vi "Panorama Generation- cameras.vi"() -> ()   [LabVIEW 2023]
uses:
  <vilib>/vision/Image Controls.llb/IMAQ Image.ctl
  <vilib>/userDefined/High Color/IMAQdx.ctl
  <vilib>/vision/driver/IMAQdx.llb/IMAQdx Acquisition Mode.ctl
  <vilib>/vision/Calibration.llb/Distortion Model.ctl
  <vilib>/vision/Calibration.llb/Distortion Model Types.ctl
  <vilib>/vision/driver/IMAQdx.llb/IMAQdx Buffer Number Mode.ctl
  <vilib>/vision/EDVR.llb/IMAQ ImageToEDVR 2D SGL.vi
  <vilib>/vision/EDVR.llb/IMAQ ImageToEDVR 2D U8.vi
  <vilib>/vision/NI_Vision_Development_Module.lvlib
  <vilib>/vision/driver/NI_Vision_Acquisition_Software.lvlib
panel:
  in  "?":T1(tab)
  in  "?":enum32{"Processing Time  Display Tab"}(tab)
  out "SSIM Flat":dbl
  out "SSIM Original":dbl
  out "Correction":dbl
  out "Flat Fielding":dbl
  out "ROI Blending":dbl
  out "Processed FPS":dbl
  in  "Stop":bool
  out "Original Luma?":bool
  out "Left corrected, adjusted, and wrapped image":T2(plugin-control) caption="Thresholded Grid"
  out "Right corrected, adjusted, and wrapped image":T2(plugin-control) caption="Thresholded Grid"
  out "Right Sample":T2(plugin-control) caption="Thresholded Grid"
  out "Left Sample":T2(plugin-control) caption="Thresholded Grid"
  out "Panorama Image":T2(plugin-control)
  in  "?":enum32{"Tunning Control Tab"}(tab)
  in  "Wrapping Factor":i32=5
  in  "Correction Interpolation":u32(ring) items=["Zero Order", "Bi-Linear", "Quadratic", "Cubic Spline"]
  in  "Grid Path":path
  in  "Blending Method":enum16{"WA", "MBB", "WE"}(ring)
  in  "Grid Name":string="grid.png"
  in  "ROI_X":i32=10
  in  "Camera 1":T3
  in  "Camera 2":T3
  out "Right corrected, adjusted, and wrapped grid":T2(plugin-control) caption="Right  corrected wrapped grid"
  out "Left corrected, adjusted, and wrapped grid":T2(plugin-control) caption="Left corrected  and wrapped grid"
  out "Thresholded and filtered grid":T2(plugin-control) caption="Thresholded Grid"
  out "Grid Image":T2(plugin-control) caption="Circular Dotted Grid"
  out "ROI_L":T2(plugin-control)
  out "ROI_R":T2(plugin-control)
  out "Blended ROI":T2(plugin-control)
  out "Wrapped Y":i32
  out "Grid X":i32
  out "Grid Y":i32
  out "corrected":T2[](array[typedef])
  out "Adjusted":T2[](array[typedef])
  out "RGB Left":T2[](array[typedef])
  out "RGB Right":T2[](array[typedef])
  out "Y0":dbl
  out "X0":dbl
  out "Y1":dbl
  out "X1":dbl
  out "Y2":dbl
  out "X2":dbl
  out "Wrapped X":i32
  out "GP":T2[][](array[typedef])
  out "LP":T2[][](array[typedef])
  out "Masked RGB Right MBB":T2[](array[typedef])
  out "Masked RGB Left MBB":T2[](array[typedef])
  out "Combined Laplace":T2[][](array[typedef])
  out "Start Time":dbl
  out "Correction End Time":dbl
  out "Flat Fielding End Time":dbl
  out "Blending End Time":dbl
  out "Wrapped":T2[](array[typedef])
  out "error out":errorcluster
  out "corrected size":cluster{"X Resolution":i32, "Y Resolution":i32}
  # "This VI meticulously generates panoramic images through a carefully structured process:\n\nLens Distortion Correction: Specifically addressing Barrel Distortion to ensure precise visual accuracy.\nBrightness Variation Compensation: Achieving a seamless transition by compensating variations in brightness.\nROI Blending: Merging carefully determined Regions of Interest (ROIs) using a selected method (Weighted Average - Default, Multi-Band Blending, Wavelet Extraction).\nFinal Panorama Output: Projecting the corrected and blended elements to produce the ultimate panorama.\n\nUser Steps: Navigate to the \"Tuning Control Tab\" and follow these steps:\n\nSelect Grid Image Path: Specify the path for the grid image.\nInput Grid Image Name: Enter the grid image name as saved in the device, including its extension.\nChoose Left and Right Cameras: Indicate the cameras for the left and right images.\nCorrection Interpolation Type: Determine the interpolation type for the correction process (Zero-Order, or Bilinear).\nSet Wrapping Factor: Define the wrapping factor based on the angle between the cameras.\nROI Resolution: Specify the resolution for the Regions of Interest (ROIs).\nBlending Method: Select the preferred blending method (Weighted Average - Default, Multi-Band Blending, Wavelet Extraction).\nRun the VI."
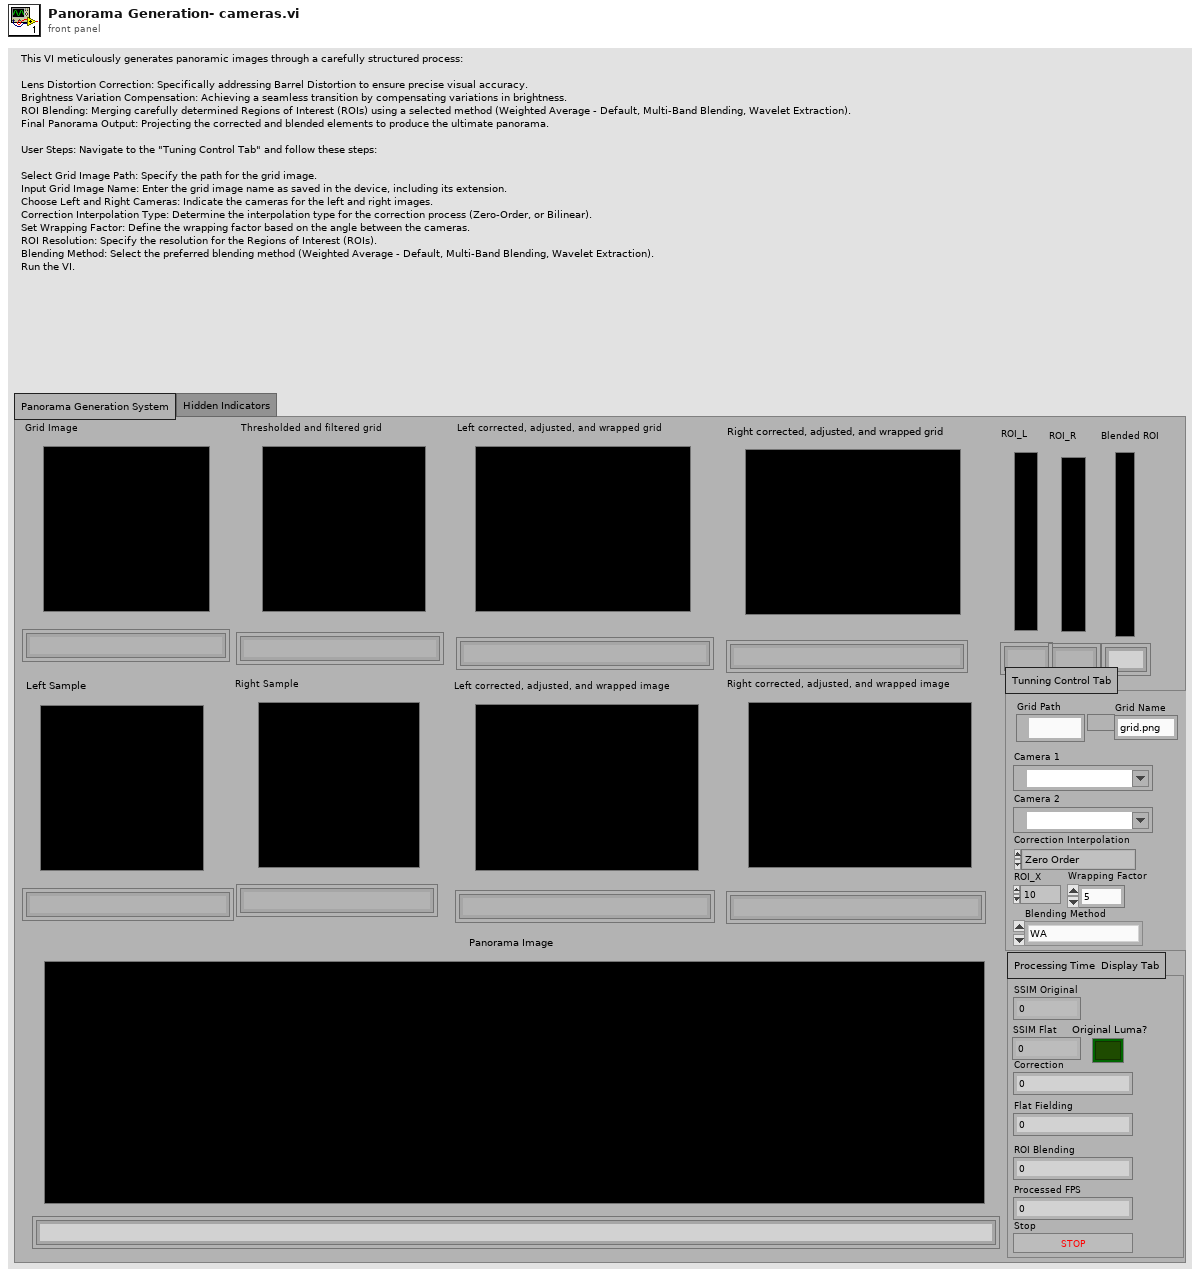
[diagram p1: front panel]
types:
  T1 = enum32{"Panorama Generation System", "Hidden Indicators"}
  T2 = typedef "IMAQ Image.ctl" = refnum<image>
  T3 = typedef "IMAQdx.ctl" = refnum<k21>
  T4 = typedef "NI_Vision_Acquisition_Software.lvlib/IMAQdx Acquisition Mode.ctl" = enum32{"One Shot", "Continuous"}
  T5 = typedef "Image Unit" = enum32{"Undefined", "Angström", "Micrometer", "Millimeter", "Centimeter", "Meter", "Kilometer", "Microinch", "Inch", "Feet", "Nautical miles", "Standard miles", "Steps"}
  T6 = typedef "Particle Parameters" = i32
  T7 = cluster{"Measurement Parameter":T6, "Range Lower Value":dbl, "Range Upper Value":dbl, "Range":bool, "Measurement Type":bool}[]
  T8 = cluster{"Corrected Image Scaling":u32, "Corrected Image Learn ROI":u32, "Learn Correction Table?":bool}
  T9 = typedef "Distortion Model.ctl" = cluster{"Distortion Model":T10, "Polynomial Model Setup":cluster{"Radial Coefficient":u32, "Tangential Coefficients ":bool}}
  T10 = typedef "Distortion Model Types.ctl" = i32
  T11 = typedef "Image Type" = u32
  T12 = typedef "Calibration Reference Points.ctl" = cluster{"Pixel Coordinates":cluster{"X":dbl, "Y":dbl}[], "Real World Coordinates":cluster{"X":dbl, "Y":dbl}[], "Unit":T5, "Image Size":cluster{"X":u32, "Y":u32}}
  T13 = cluster{cluster{"element":dbl, "element":dbl}[], cluster{"element":dbl, "element":dbl}[], "Unit":T5, cluster{"X Resolution":i32, "Y Resolution":i32}}
  T14 = typedef "NI_Vision_Acquisition_Software.lvlib/IMAQdx Buffer Number Mode.ctl" = enum32{"Next", "Last", "Buffer Number", "Every", "Last New"}
  T15 = cluster{"Model":i32, "corrected size":cluster{"X Resolution":i32, "Y Resolution":i32}, "Polynomial Degree":i32}
  T16 = cluster{"Estimate Background?":bool, "Method":i32, "Polynomial Degree":i32, "corrected size":cluster{"X Resolution":i32, "Y Resolution":i32}, "Niblack Deviation Factor (0.2)":dbl}
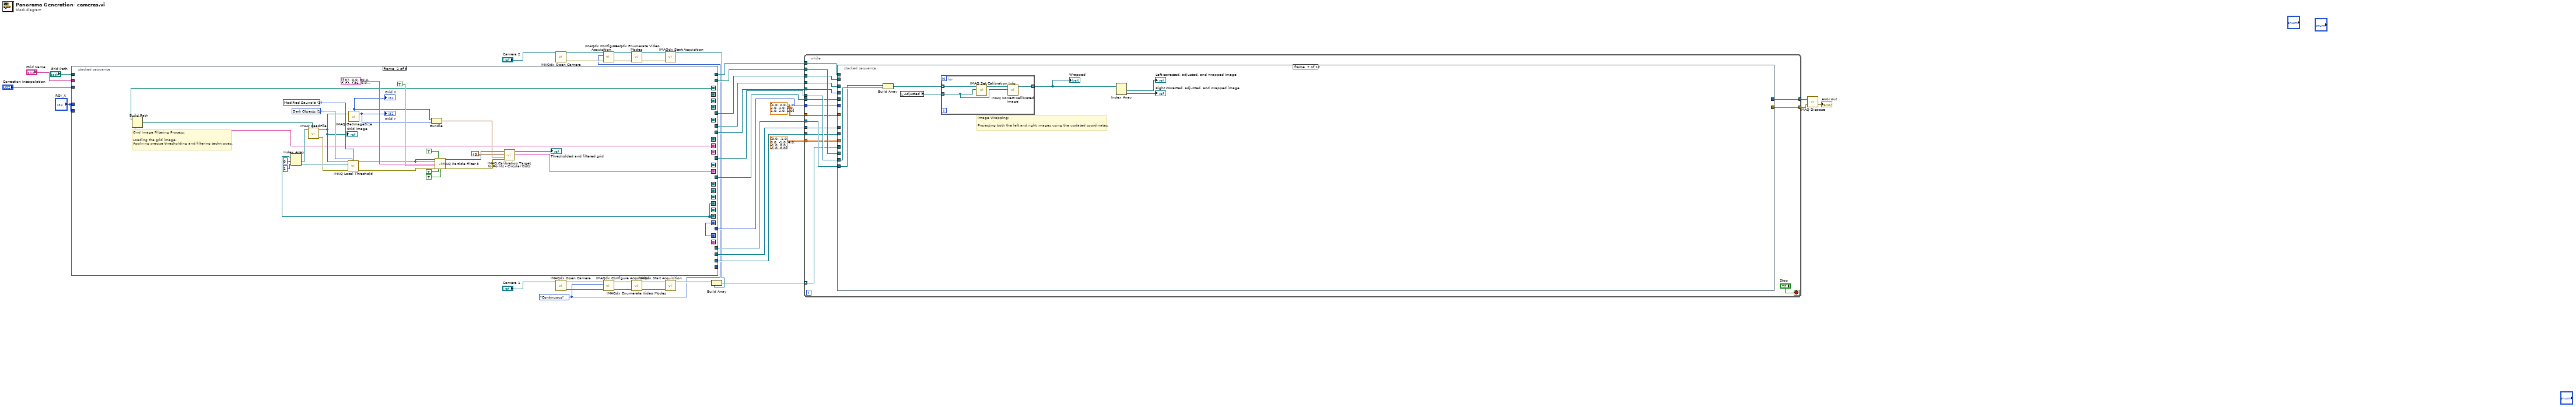
[diagram p0: block diagram]
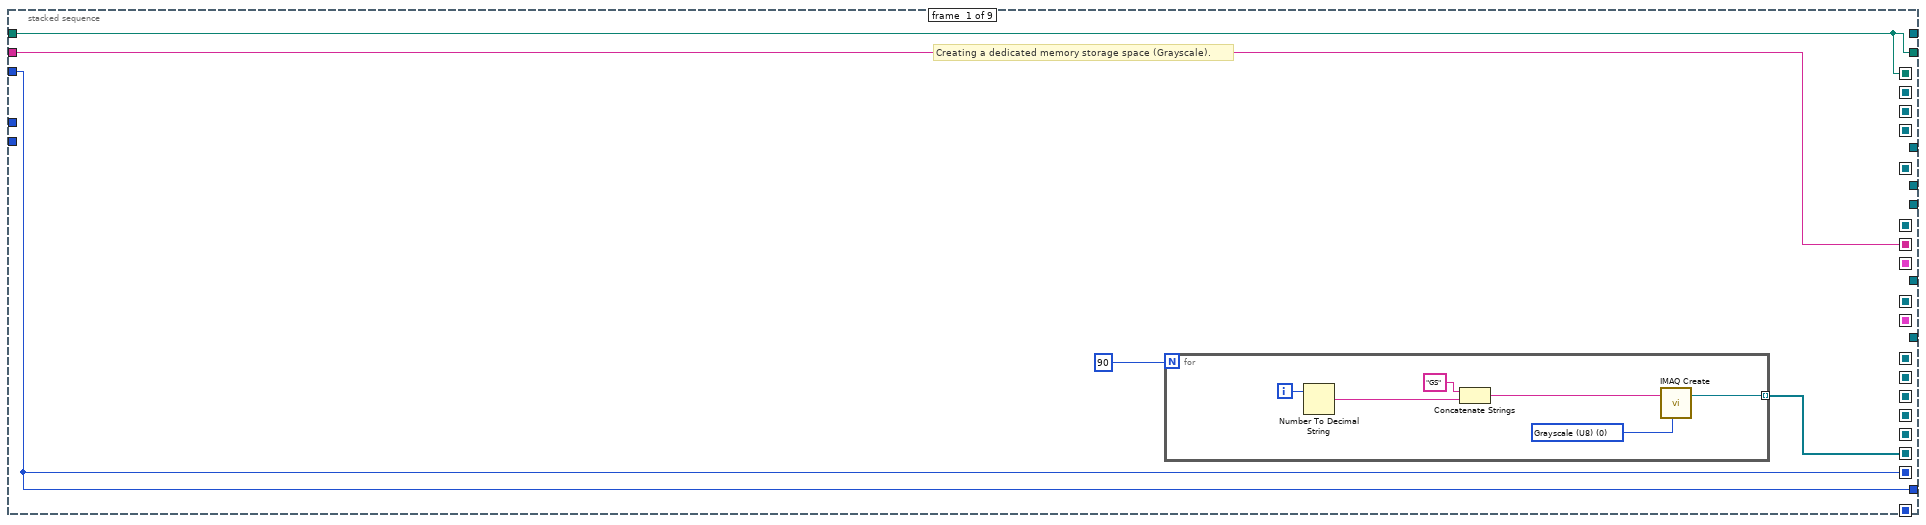
[diagram p2: hidden frame]
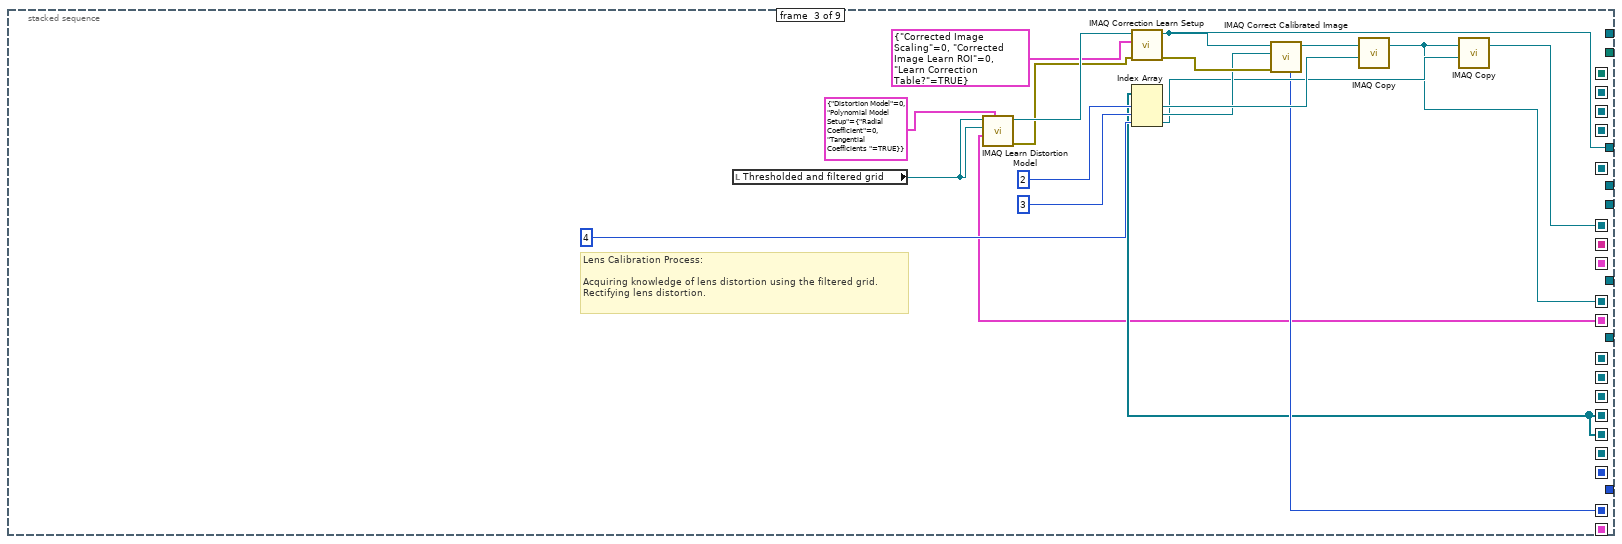
[diagram p3: hidden frame]
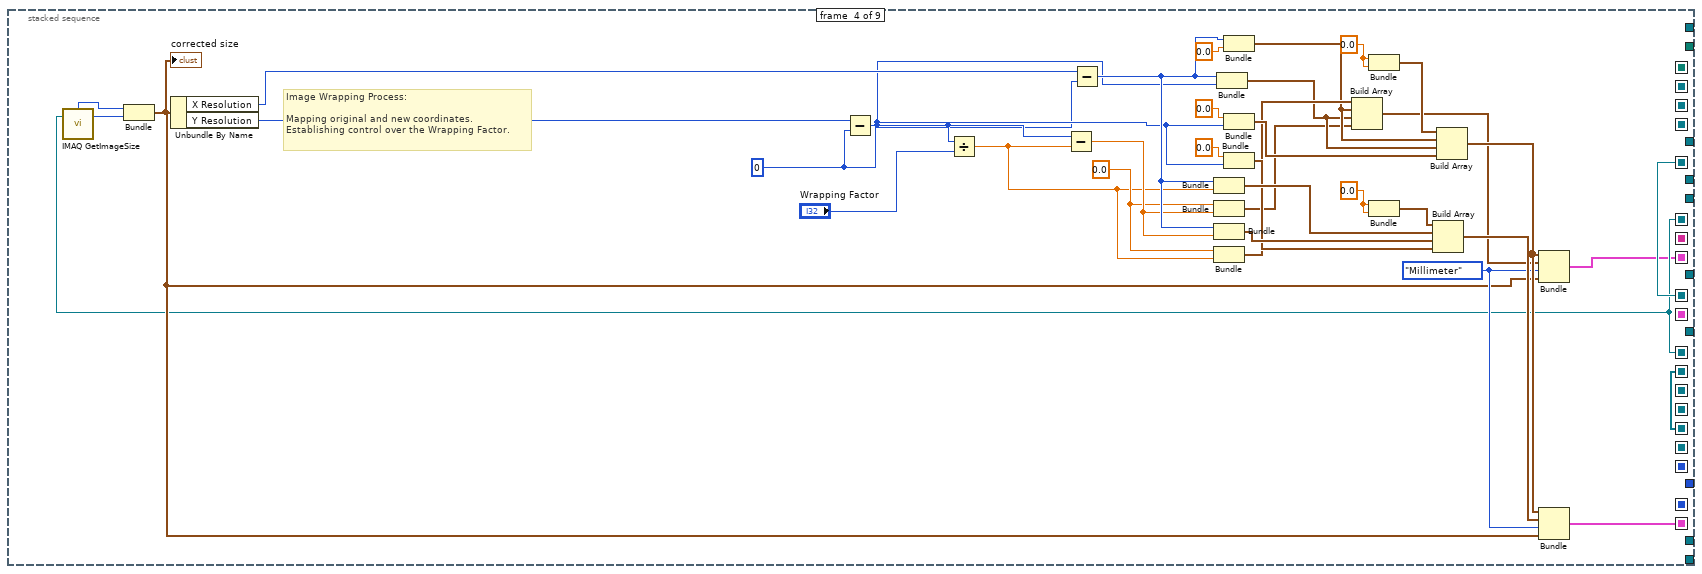
[diagram p4: hidden frame]
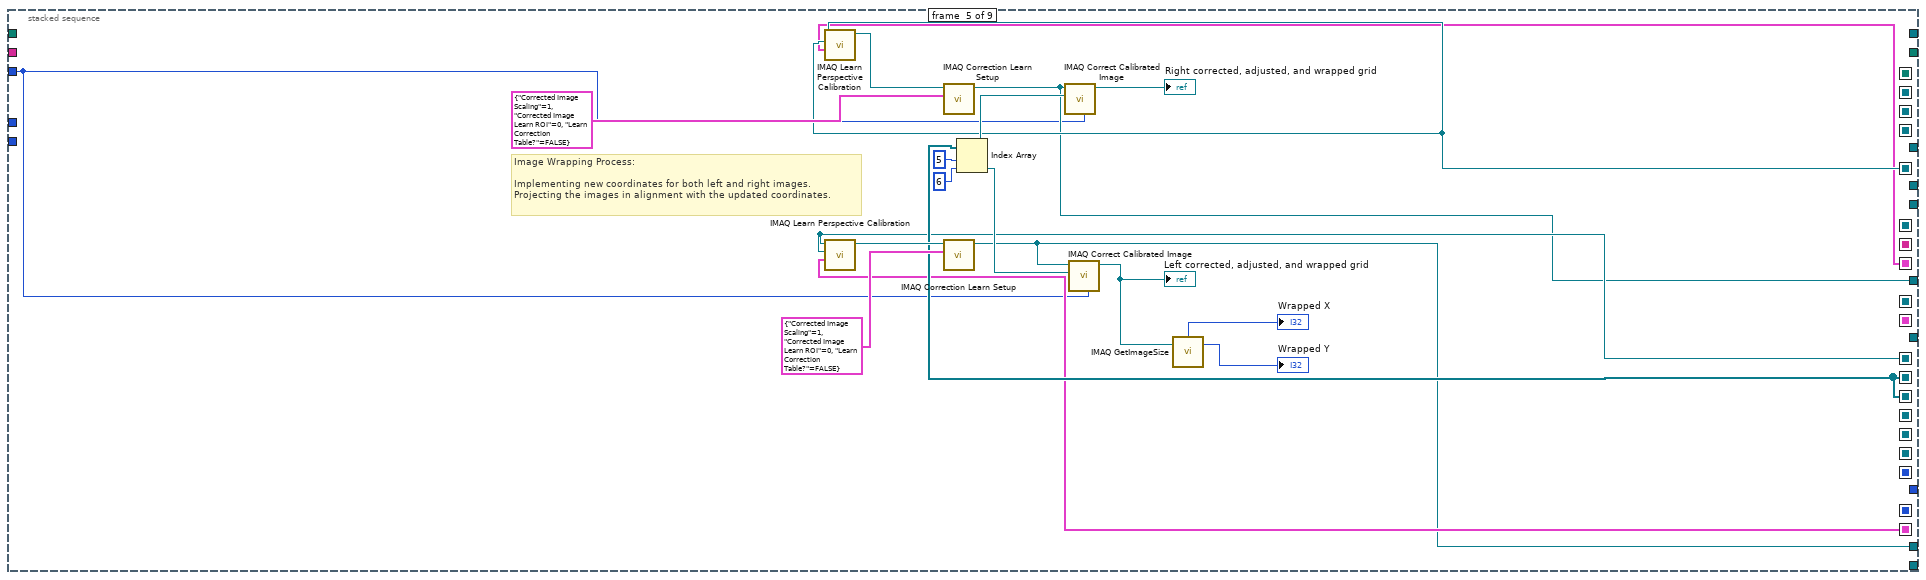
[diagram p5: hidden frame]
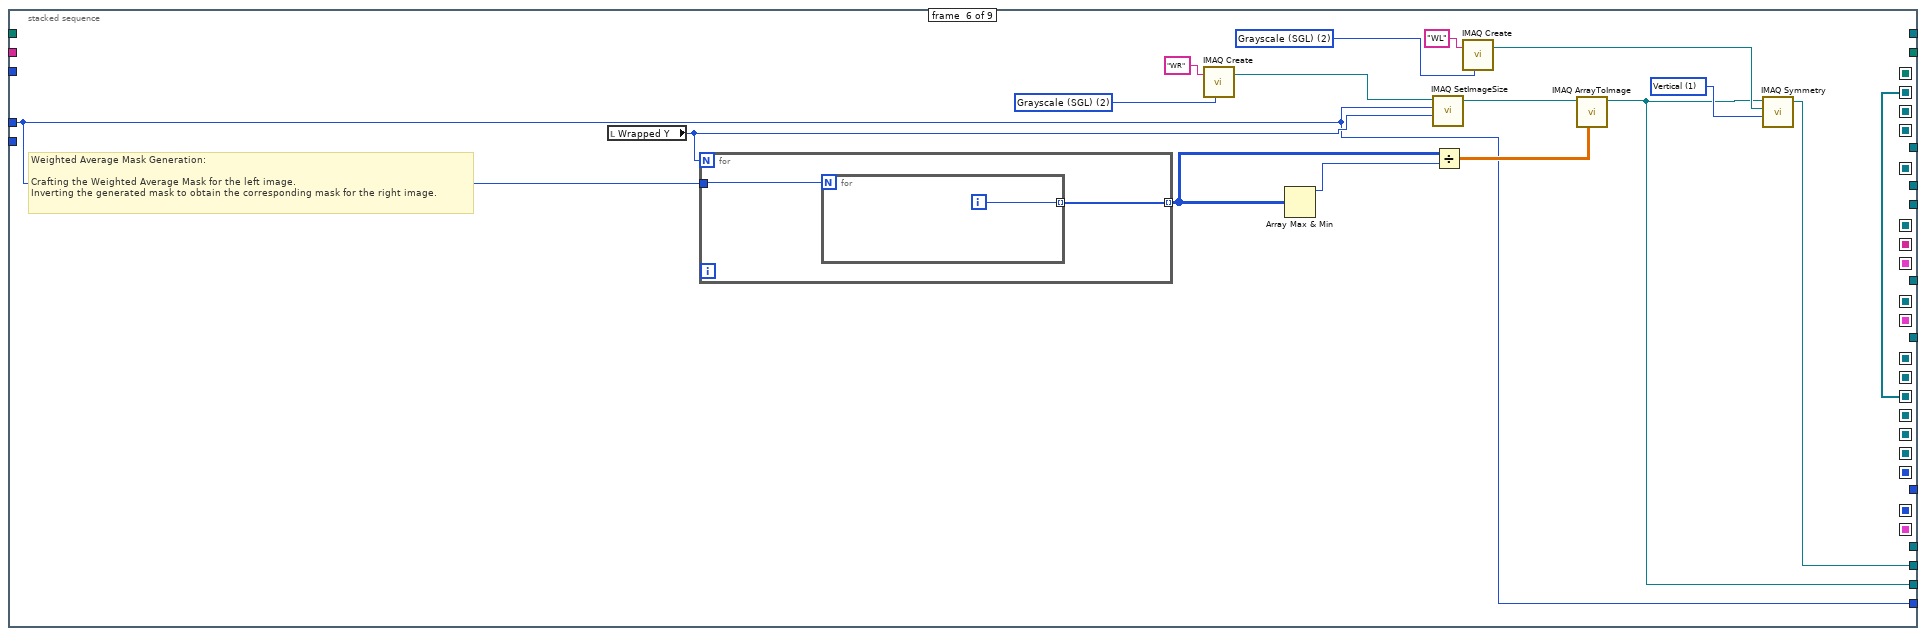
[diagram p6: hidden frame]
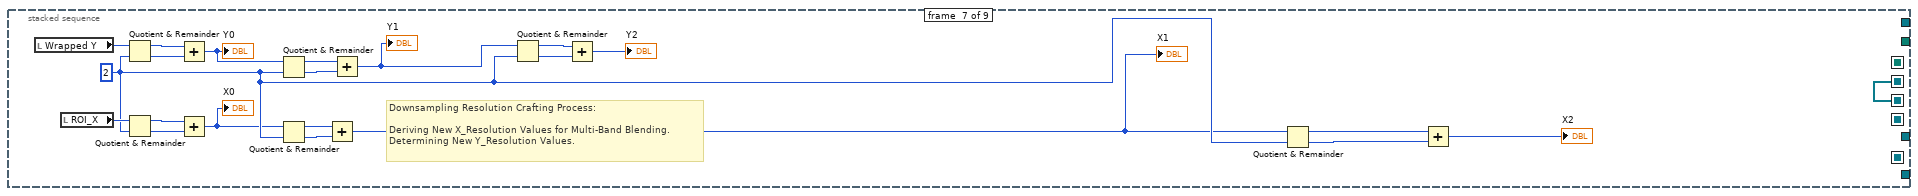
[diagram p7: hidden frame]
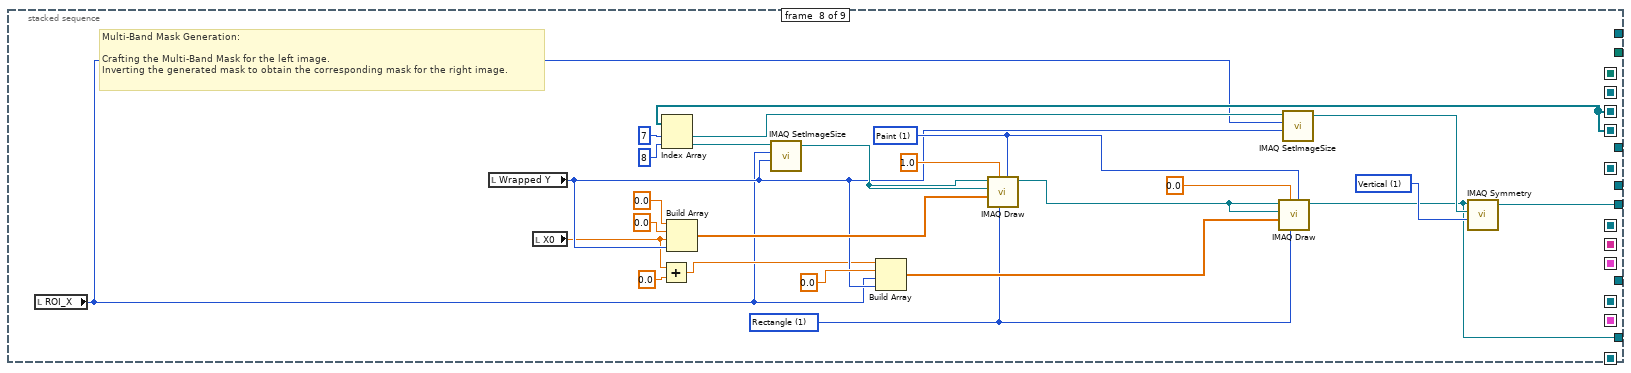
[diagram p8: hidden frame]
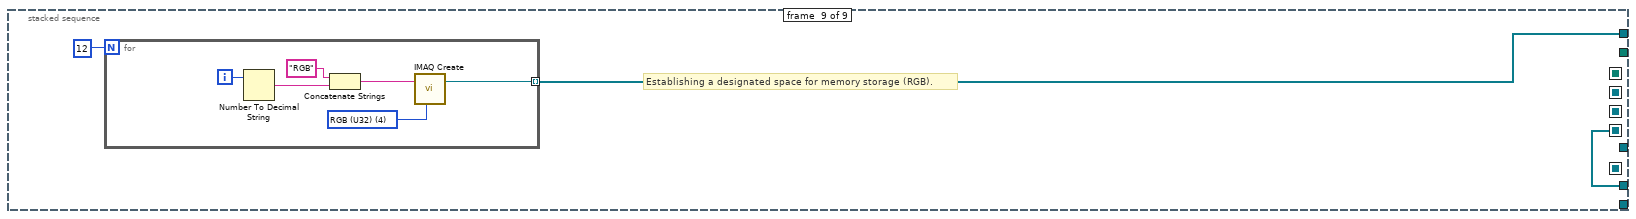
[diagram p9: hidden frame]
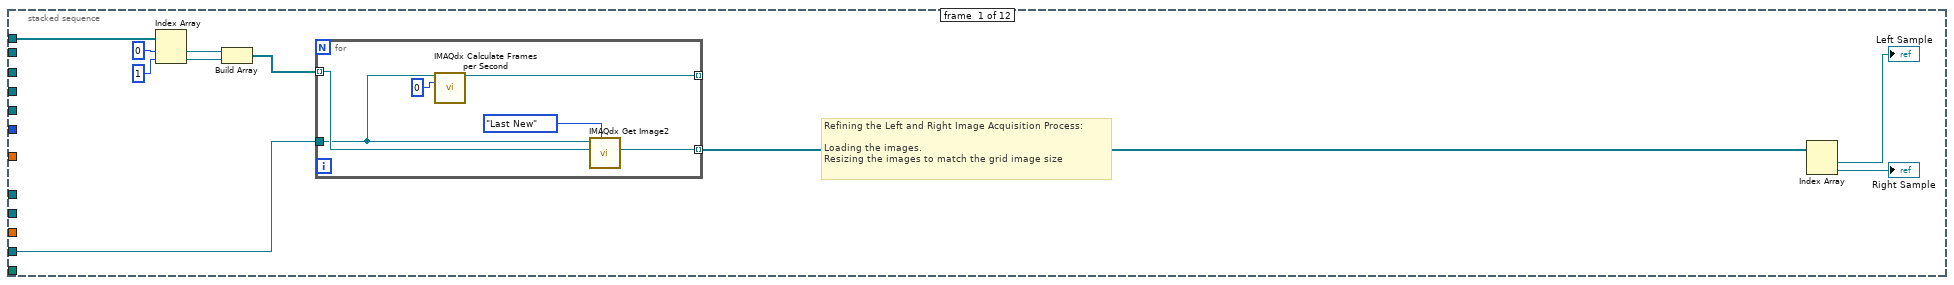
[diagram p10: hidden frame]
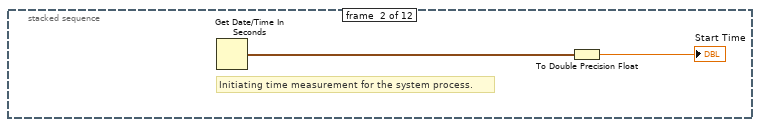
[diagram p11: hidden frame]
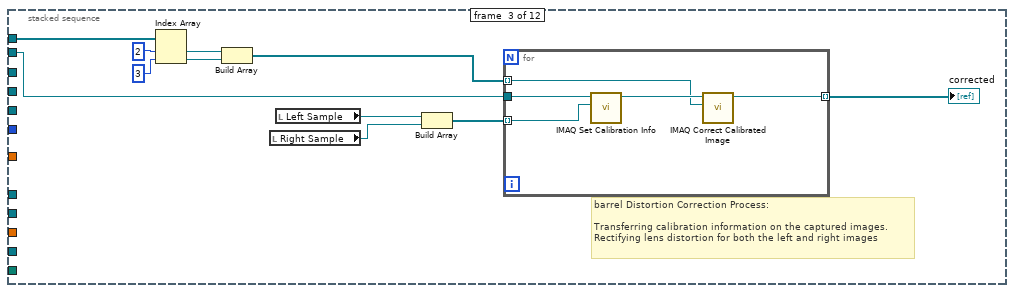
[diagram p12: hidden frame]
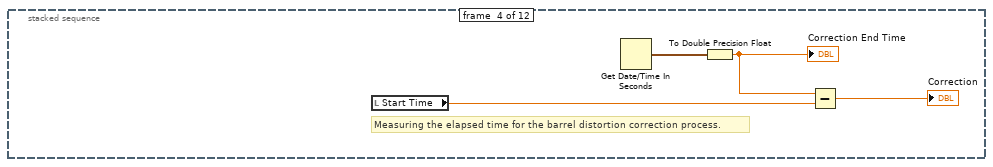
[diagram p13: hidden frame]
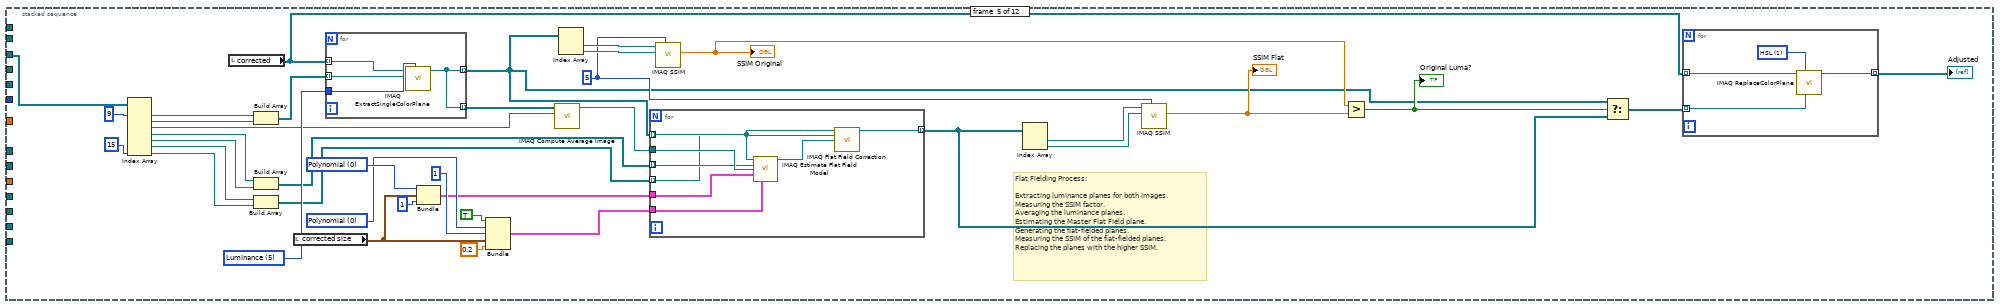
[diagram p14: hidden frame]
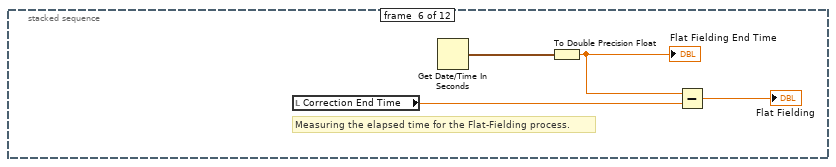
[diagram p15: hidden frame]
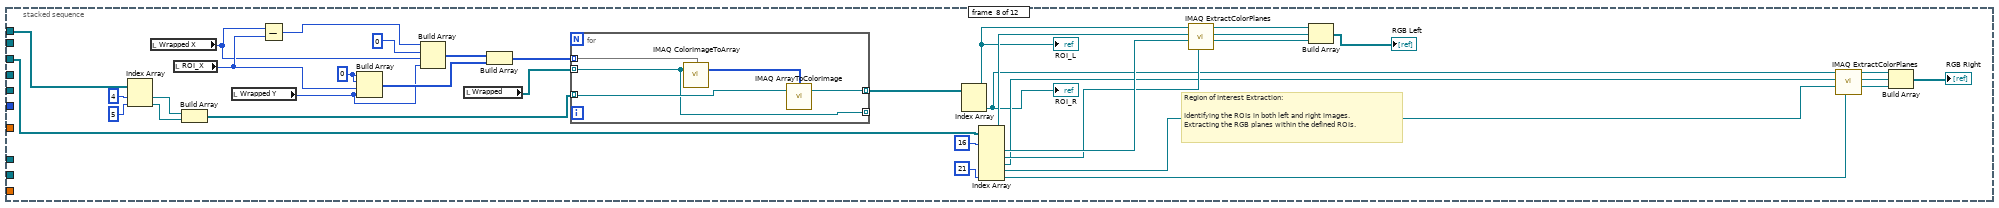
[diagram p16: hidden frame]
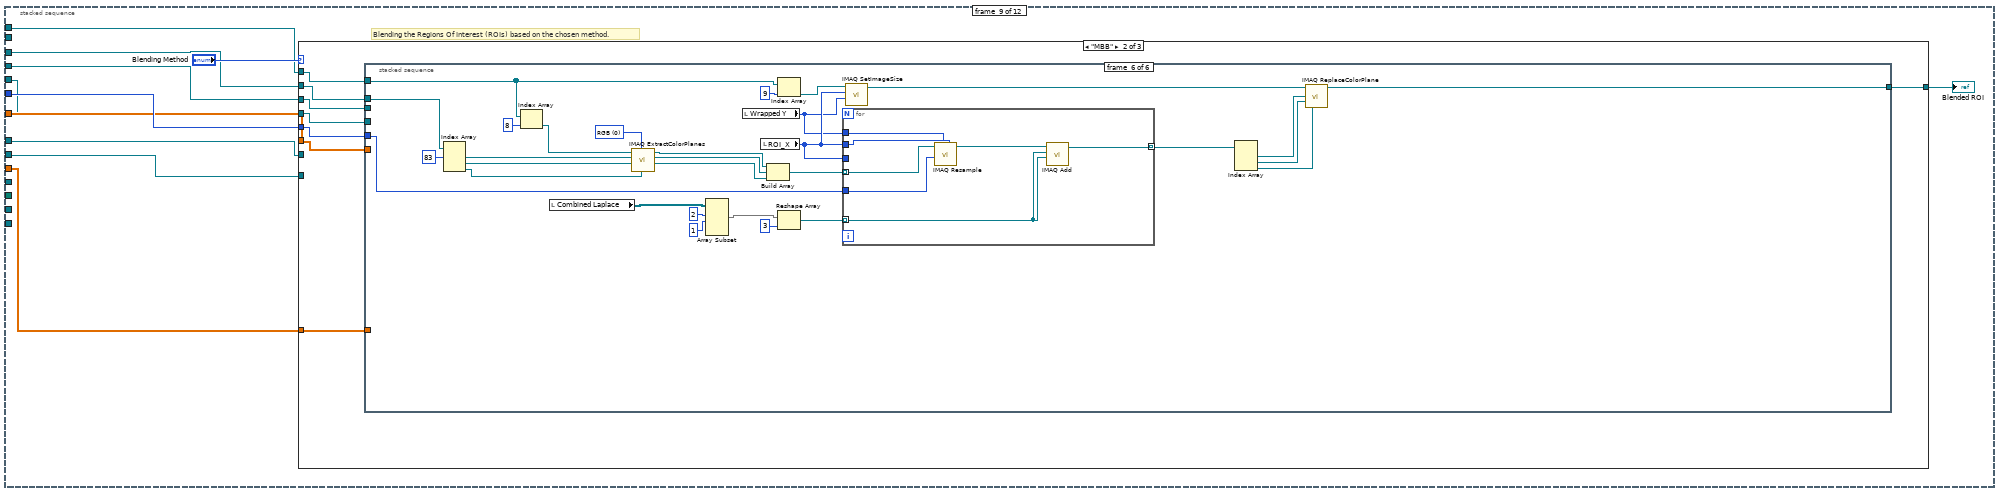
[diagram p17: hidden frame]
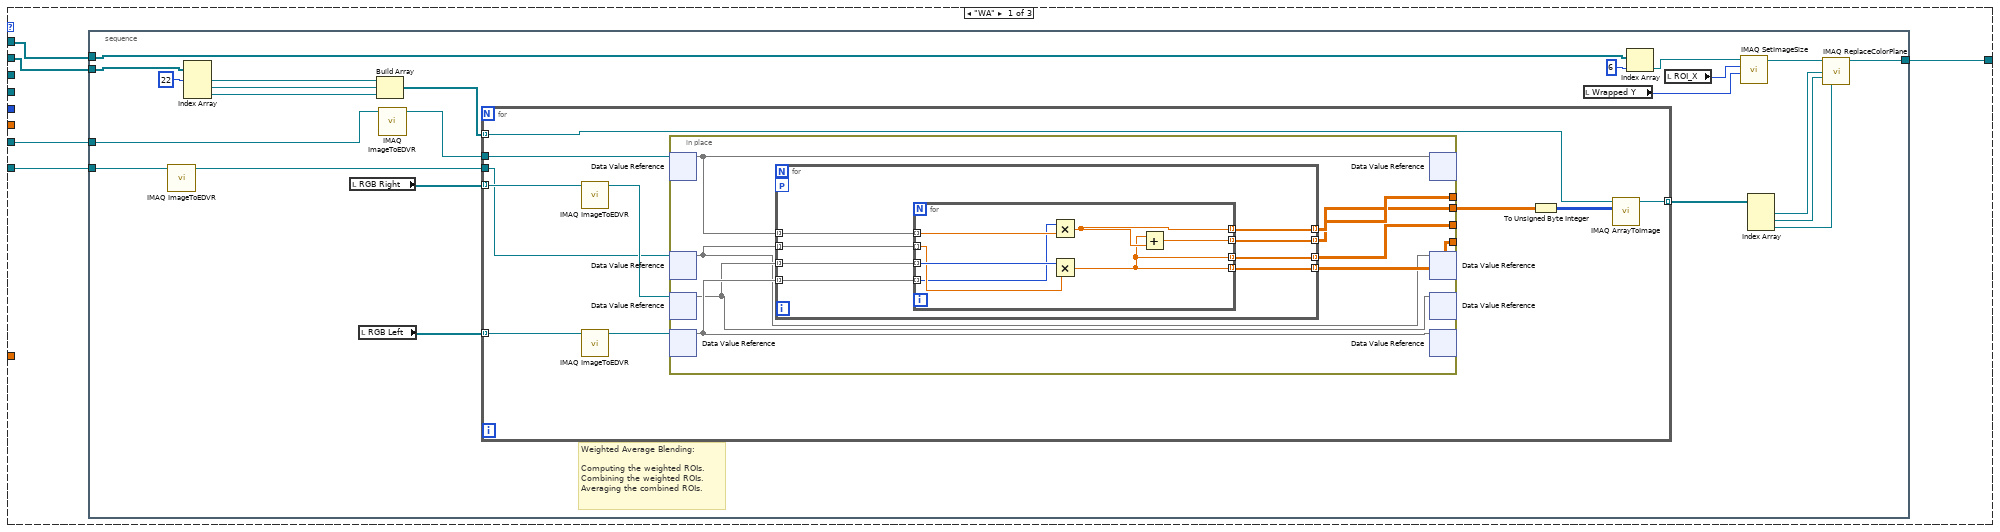
[diagram p18: hidden frame]
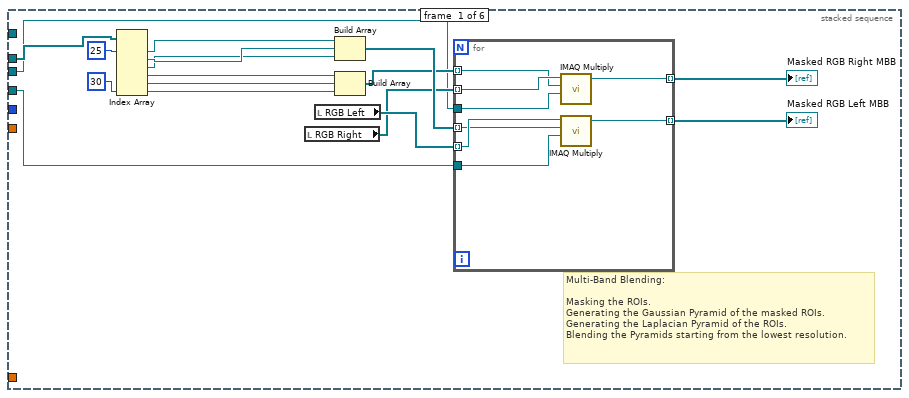
[diagram p19: hidden frame]
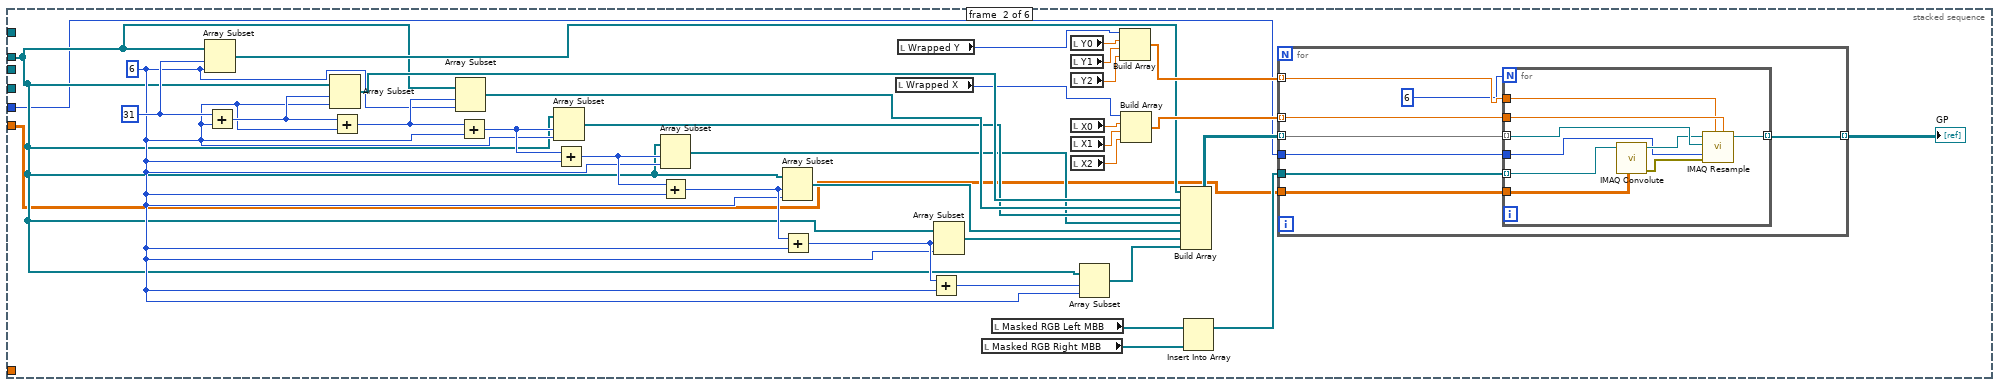
[diagram p20: hidden frame]
diagram:
  w2 = IMAQdx_Acquisition_Mode."Continuous" ("Continuous?")
  n1 = stacked-sequence {
    seq-local: [w40 _ _ _ _ _ _ _ _] -> [_ w56 _ _ _ _ _ _ _]
    seq-local: [w42 _ _ _ _ _ _ _ _] -> [_ w55 _ _ _ _ _ _ _]
    seq-local: [w39 _ _ _ _ _ _ _ _] -> [_ w54 _ _ _ _ _ _ _]
    seq-local: [w41 _ _ _ _ _ _ _ _] -> [_ w53 _ _ _ _ _ _ _]
    seq-local: [_ w54 _ _ _ _ _ _ _] -> [_ _ w83 _ _ _ _ _ _]
    seq-local: [_ w53 _ _ _ _ _ _ _] -> [_ _ w82 _ _ _ _ _ _]
    seq-local: [_ w50 _ _ _ _ _ _ _] -> [_ _ w78 _ _ _ _ _ _]
    seq-local: [_ _ w82 _ _ _ _ _ _] -> [_ _ _ w105 _ _ _ _ _]
    seq-local: [_ _ w81 _ _ _ _ _ _] -> [_ _ _ w104 _ _ _ _ _]
    seq-local: [_ _ w80 _ _ _ _ _ _] -> [_ _ _ w100 _ _ _ _ _]
    seq-local: [_ _ _ w105 _ _ _ _ _] -> [_ _ _ _ w140 _ _ _ _]
    seq-local: [_ _ _ w104 _ _ _ _ _] -> [_ _ _ _ w139 _ _ _ _]
    seq-local: [_ _ _ w100 _ _ _ _ _] -> [_ _ _ _ w138 _ _ _ _]
    seq-local: [_ _ _ w99 _ _ _ _ _] -> [_ _ _ _ w137 _ _ _ _]
    seq-local: [_ _ _ w98 _ _ _ _ _] -> [_ _ _ _ w136 _ _ _ _]
    seq-local: [_ _ _ _ w140 _ _ _ _] -> [_ _ _ _ _ w156 _ _ _]
    seq-local: [_ _ _ _ _ w156 _ _ _] -> [_ _ _ _ _ _ w172 _ _]
    seq-local: [_ _ _ _ _ _ w172 _ _] -> [_ _ _ _ _ _ _ w197 _]
    seq-local: [_ _ _ _ _ _ _ w197 _] -> [_ _ _ _ _ _ _ _ w221]
    tunnel: "Grid Path" -> [w40 _ _ _ _ _ _ _ _]
    tunnel: "Grid Name" -> [w42 _ _ _ _ _ _ _ _]
    tunnel: "Correction Interpolation" -> [w39 _ _ _ w133 _ _ _ _]
    tunnel: [_ _ w79 _ _ _ _ _ _] -> w28
    tunnel: [_ _ _ _ w135 _ _ _ _] -> w26
    tunnel: [_ _ _ _ w134 _ _ _ _] -> w27
    tunnel: [_ _ _ _ _ _ _ w196 _] -> w24
    tunnel: [_ _ _ _ _ _ _ w195 _] -> w25
    tunnel: [_ _ _ _ _ _ _ _ w221] -> w30
    tunnel: [_ _ _ _ _ _ _ _ w219] -> w29
    tunnel: [_ _ _ _ _ w155 _ _ _] -> w23
    tunnel: [_ _ _ _ _ w154 _ _ _] -> w22
    tunnel: [w40 _ _ _ _ _ _ _ _] -> w21
    tunnel: [w39 _ _ _ _ _ _ _ _] -> w20
    tunnel: "ROI_X" -> [_ _ _ _ _ _ _ _ _]
    tunnel: "ROI_X" -> [_ _ _ _ _ w153 _ _ _]
    tunnel: [_ _ _ _ _ w153 _ _ _] -> _
    frame #0 {
      # "Creating a dedicated memory storage space (Grayscale)."
      n2 = for {
        N: 90 -> [_]
        tunnel: [w44] -> w41 mode=indexing
        i -> [w45]
        w46 = T11 0 items=["Grayscale (U8)", "Grayscale (I16)", "Grayscale (SGL)", "Complex (CSG)", "RGB (U32)", "HSL (U32)", "RGB (U64)", "Grayscale (U16)"] ("Image Type")
        n3 = Number To Decimal String(number=w45) -> (decimal integer string=w49:string)  [unwired: 1 out]
        n4 = Concatenate Strings("GS" ("string"), w49) -> (w48:string)
        n5 = call "IMAQ Create"("Image Name"=w48, "Image Type"=w46) -> ("New Image"=w44:T2)  [unwired: 2 in, 2 out]
      }
    }
    frame #1 {
      w69 = u32 3 items=["Niblack", "Background Correction", "Sauvola", "Modified Sauvola"] ("Method (Niblack)")
      w70 = u32 1 items=["Bright Objects", "Dark Objects"] ("Look For (Bright Objects)")
      # "Grid Image Filtering Process:\n\nLoading the grid image.\nApplying precise thresholding and filtering techniques."
      n6 = Build Path(base path=w56, name or relative path=w55) -> (appended path=w77:path)
      n7 = Index Array(array=w53, index #1=0 ("index"), index #2=1 ("index")) -> (element #1=w67:T2, element #2=w66:T2)
      n8 = call "IMAQ ReadFile"("File Path"=w77, "Image"=w67) -> ("error out"=w57:errorcluster, "Image Out"=w58:T2)  [unwired: 3 in, 5 out]
      "Grid Image" <- w58
      n9 = call "IMAQ Local Threshold"("Image Src"=w58, "Look For (Bright Objects)"=w70, "Method (Niblack)"=w69, "Image Dst"=w66, "error in (no error)"=w57) -> ("Image Dst Out"=w64:T2, "error out"=w76:errorcluster)  [unwired: 9 in]
      n10 = call "IMAQ GetImageSize"("Image"=w58) -> ("Y Resolution"=w51:i32, "X Resolution"=w52:i32)  [unwired: 3 in, 1 out]
      "Grid X" <- w52
      "Grid Y" <- w51
      n11 = Bundle("X Resolution"=w52, "Y Resolution"=w51) -> (w59:cluster{"X Resolution":i32, "Y Resolution":i32})  [unwired: 1 in]
      n12 = call "IMAQ Particle Filter 3"("Image Src"=w64, "Connectivity 4/8 (8)"=TRUE, "Image Dst"=w64, "Selection Values"=T7 [{"Measurement Parameter"=37, "Range Lower Value"=0.0, "Range Upper Value"=50.0, "Range"=FALSE, "Measurement Type"=FALSE}, {"Measurement Parameter"=36, "Range Lower Value"=0.0, "Range Upper Value"=0.0, "Range"=FALSE, "Measurement Type"=FALSE}], "Keep/Remove Particles (F)"=TRUE, "error in (no error)"=w76, "Reject Border? (F)"=TRUE, "Fill Holes? (F)"=TRUE) -> ("Image Dst Out"=w60:T2, "error out"=w61:errorcluster)  [unwired: 1 in, 5 out]
      n13 = call "IMAQ Calibration Target to Points - Circular Dots"("error in (no error)"=w61, "Grid Size"=w59, "Grid Descriptor"=cluster{"X Step":sgl, "Y Step":sgl, "Unit":T5} {"X Step"=3.6, "Y Step"=3.6, "Unit"=enum."Millimeter"}, "Target Image"=w60) -> ("Reference Points"=w50:T12, "Target Image (dup)"=→"Thresholded and filtered grid":T2)  [unwired: 5 in, 1 out]
    }
    frame #2 {
      # "Lens Calibration Process:\n\nAcquiring knowledge of lens distortion using the filtered grid.\nRectifying lens distortion."
      n14 = local read "Thresholded and filtered grid"() -> (w87:T2)
      n15 = call "IMAQ Learn Distortion Model"("Distortion Model Setup"=T9 {"Distortion Model"=0, "Polynomial Model Setup"={"Radial Coefficient"=0, "Tangential Coefficients "=TRUE}}, "Reference Points"=w78, "Image"=w87, "Calibration Template Image"=w87) -> ("error out"=w94:errorcluster, "Calibration Template Image Out"=w95:T2)  [unwired: 6 in]
      n16 = call "IMAQ Correction Learn Setup"("error in (no error)"=w94, "Correction Learn Setup"=T8 {"Corrected Image Scaling"=0, "Corrected Image Learn ROI"=0, "Learn Correction Table?"=TRUE}, "Calibration Template Image"=w95) -> ("error out"=w93:errorcluster, "Calibration Template Image Out"=w79:T2)  [unwired: 7 in]
      n17 = Index Array(array=w82, index #1=2 ("index"), index #2=3 ("index"), index #3=4 ("index")) -> (element #1=w88:T2, element #2=w86:T2, element #3=w85:T2)
      n18 = call "IMAQ Correct Calibrated Image"("Interpolation Type"=w83, "error in (no error)"=w93, "Image Dst"=w86, "Image Src"=w79) -> ("Corrected Image"=w96:T2)  [unwired: 6 in, 1 out]
      n19 = call "IMAQ Copy"("Image Dst"=w88, "Image Src"=w96) -> ("Image Dst Out"=w81:T2)  [unwired: 4 in, 1 out]
      n20 = call "IMAQ Copy"("Image Dst"=w85, "Image Src"=w81) -> ("Image Dst Out"=w80:T2)  [unwired: 4 in, 1 out]
    }
    frame #3 {
      w114 = 0.0 ("element")
      w112 = 0 ("y")
      w110 = 0.0 ("element")
      w107 = 0.0 ("element")
      w113 = Image_Unit."Millimeter" ("Unit")
      # "Image Wrapping Process:\n\nMapping original and new coordinates.\nEstablishing control over the Wrapping Factor."
      n21 = call "IMAQ GetImageSize"("Image"=w100) -> ("Y Resolution"=w103:i32, "X Resolution"=w102:i32)  [unwired: 3 in, 1 out]
      n22 = Bundle("X Resolution"=w102, "Y Resolution"=w103) -> (w101:cluster{"X Resolution":i32, "Y Resolution":i32})  [unwired: 1 in]
      "corrected size" <- w101
      n23 = Unbundle By Name(w101) -> ("X Resolution"=w125:i32, "Y Resolution"=w124:i32)
      n24 = Subtract(x=w124, y=w112) -> (x-y=w121:i32)
      n25 = Divide(x=w121, y="Wrapping Factor") -> (x/y=w106:dbl)
      n26 = Subtract(x=w121, y=w106) -> (x-y=w117:dbl)
      n27 = Subtract(x=w125, y=w112) -> (x-y=w122:i32)
      n28 = Bundle(w122, w106) -> (w129:cluster{i32, dbl})  [unwired: 1 in]
      n29 = Bundle("element"=w114, w117) -> (w116:cluster{"element":dbl, dbl})  [unwired: 1 in]
      n30 = Bundle(w122, w117) -> (w128:cluster{i32, dbl})  [unwired: 1 in]
      n31 = Bundle("element"=w114, w106) -> (w120:cluster{"element":dbl, dbl})  [unwired: 1 in]
      n32 = Bundle(w122, w121) -> (w118:cluster{i32, i32})  [unwired: 1 in]
      n33 = Bundle(w122, "element"=0.0) -> (w119:cluster{i32, "element":dbl})  [unwired: 1 in]
      n34 = Bundle("element"=0.0, w121) -> (w131:cluster{"element":dbl, i32})  [unwired: 1 in]
      n35 = Bundle("element"=0.0, w121) -> (w127:cluster{"element":dbl, i32})  [unwired: 1 in]
      n36 = Build Array(w120, w119, w118, w116) -> (w115:cluster{"element":dbl, "element":dbl}[])
      n37 = Bundle("element"=w107, "element"=w107) -> (w132:cluster{"element":dbl, "element":dbl})  [unwired: 1 in]
      n38 = Bundle("element"=w110, "element"=w110) -> (w130:cluster{"element":dbl, "element":dbl})  [unwired: 1 in]
      n39 = Build Array(w130, w129, w128, w127) -> (w126:cluster{"element":dbl, "element":dbl}[])
      n40 = Build Array(w132, w119, w118, w131) -> (w123:cluster{"element":dbl, "element":dbl}[])
      n41 = Bundle(w123, w115, "Unit"=w113, w101) -> (w99:T13)  [unwired: 1 in]
      n42 = Bundle(w123, w126, "Unit"=w113, w101) -> (w98:T13)  [unwired: 1 in]
    }
    frame #4 {
      # "Image Wrapping Process:\n\nImplementing new coordinates for both left and right images.\nProjecting the images in alignment with the updated coordinates."
      n43 = call "IMAQ Learn Perspective Calibration"("Reference Points"=w137, "Image"=w139, "Calibration Template Image"=w139) -> ("Calibration Template Image Out"=w150:T2)  [unwired: 7 in, 1 out]
      n44 = call "IMAQ Learn Perspective Calibration"("Reference Points"=w136, "Image"=w138, "Calibration Template Image"=w138) -> ("Calibration Template Image Out"=w152:T2)  [unwired: 7 in, 1 out]
      n45 = call "IMAQ Correction Learn Setup"("Correction Learn Setup"=T8 {"Corrected Image Scaling"=1, "Corrected Image Learn ROI"=0, "Learn Correction Table?"=FALSE}, "Calibration Template Image"=w150) -> ("Calibration Template Image Out"=w135:T2)  [unwired: 8 in, 1 out]
      n46 = call "IMAQ Correction Learn Setup"("Correction Learn Setup"=T8 {"Corrected Image Scaling"=1, "Corrected Image Learn ROI"=0, "Learn Correction Table?"=FALSE}, "Calibration Template Image"=w152) -> ("Calibration Template Image Out"=w134:T2)  [unwired: 8 in, 1 out]
      n47 = Index Array(array=w140, index #1=5 ("index"), index #2=6 ("index")) -> (element #1=w145:T2, element #2=w144:T2)
      n48 = call "IMAQ Correct Calibrated Image"("Interpolation Type"=w133, "Image Dst"=w145, "Image Src"=w135) -> ("Corrected Image"=→"Right corrected, adjusted, and wrapped grid":T2)  [unwired: 7 in, 1 out]
      n49 = call "IMAQ Correct Calibrated Image"("Interpolation Type"=w133, "Image Dst"=w144, "Image Src"=w134) -> ("Corrected Image"=w141:T2)  [unwired: 7 in, 1 out]
      "Left corrected, adjusted, and wrapped grid" <- w141
      n50 = call "IMAQ GetImageSize"("Image"=w141) -> ("Y Resolution"=→"Wrapped Y":i32, "X Resolution"=→"Wrapped X":i32)  [unwired: 3 in, 1 out]
    }
    frame #5 {
      w161 = u32 1 items=["Horizontal", "Vertical", "Central", "1st Diagonal", "2nd Diagonal"] ("Type of Symmetry")
      w162 = T11 2 items=["Grayscale (U8)", "Grayscale (I16)", "Grayscale (SGL)", "Complex (CSG)", "RGB (U32)", "HSL (U32)", "RGB (U64)", "Grayscale (U16)"] ("Image Type")
      w165 = T11 2 items=["Grayscale (U8)", "Grayscale (I16)", "Grayscale (SGL)", "Complex (CSG)", "RGB (U32)", "HSL (U32)", "RGB (U64)", "Grayscale (U16)"] ("Image Type")
      # "Weighted Average Mask Generation:\n\nCrafting the Weighted Average Mask for the left image.\nInverting the generated mask to obtain the corresponding mask for the right image."
      n51 = local read "Wrapped Y"() -> (w160:i32)
      n52 = for {
        N: w160 -> [_]
        tunnel: [w170] -> w158 mode=indexing
        tunnel: w153 -> [w169]
        n53 = for {
          N: w169 -> [_]
          tunnel: [w171] -> w170 mode=indexing
          i -> [w171]
        }
      }
      n54 = call "IMAQ Create"("Image Name"="WR", "Image Type"=w165) -> ("New Image"=w167:T2)  [unwired: 2 in, 2 out]
      n55 = Array Max & Min(array=w158) -> (max value=w157:i32)  [unwired: 3 out]
      n56 = call "IMAQ SetImageSize"("Y Resolution"=w160, "X Resolution"=w153, "Image"=w167) -> ("Image Out"=w166:T2)  [unwired: 2 in, 1 out]
      n57 = Divide(x=w158, y=w157) -> (x/y=w159:dbl[][])
      n58 = call "IMAQ Create"("Image Name"="WL", "Image Type"=w162) -> ("New Image"=w164:T2)  [unwired: 2 in, 2 out]
      n59 = call "IMAQ ArrayToImage"("Image Pixels (Float)"=w159, "Image"=w166) -> ("Image Out"=w154:T2)  [unwired: 8 in, 1 out]
      n60 = call "IMAQ Symmetry"("Type of Symmetry"=w161, "Image Dst"=w164, "Image Src"=w154) -> ("Image Dst Out"=w155:T2)  [unwired: 2 in, 1 out]
    }
    frame #6 {
      w179 = 2 ("y")
      # "Downsampling Resolution Crafting Process:\n\nDeriving New X_Resolution Values for Multi-Band Blending.\nDetermining New Y_Resolution Values."
      n61 = local read "Wrapped Y"() -> (w192:i32)
      n62 = local read "ROI_X"() -> (w193:i32)
      n63 = Quotient & Remainder(x=w192, y=w179) -> (x-y*floor(x/y)=w189:i32, floor(x/y)=w188:i32)
      n64 = Quotient & Remainder(x=w193, y=w179) -> (x-y*floor(x/y)=w191:i32, floor(x/y)=w190:i32)
      n65 = Add(x=w189, y=w188) -> (x+y=w176:i32)
      "Y0" <- w176
      n66 = Add(x=w191, y=w190) -> (x+y=w173:i32)
      "X0" <- w173
      n67 = Quotient & Remainder(x=w176, y=w179) -> (x-y*floor(x/y)=w187:i32, floor(x/y)=w186:i32)
      n68 = Quotient & Remainder(x=w173, y=w179) -> (x-y*floor(x/y)=w185:i32, floor(x/y)=w184:i32)
      n69 = Add(x=w185, y=w184) -> (x+y=w174:i32)
      "X1" <- w174
      n70 = Add(x=w187, y=w186) -> (x+y=w177:i32)
      "Y1" <- w177
      n71 = Quotient & Remainder(x=w177, y=w179) -> (x-y*floor(x/y)=w183:i32, floor(x/y)=w182:i32)
      n72 = Add(x=w183, y=w182) -> (x+y=→"Y2":i32)
      n73 = Quotient & Remainder(x=w174, y=w179) -> (x-y*floor(x/y)=w181:i32, floor(x/y)=w180:i32)
      n74 = Add(x=w181, y=w180) -> (x+y=→"X2":i32)
    }
    frame #7 {
      w201 = u32 1 items=["Horizontal", "Vertical", "Central", "1st Diagonal", "2nd Diagonal"] ("Type of Symmetry")
      w205 = u16 1 items=["Line", "Rectangle", "Oval"] ("Shape to draw")
      w212 = u16 1 items=["Frame", "Paint", "Invert Frame", "Invert Paint"] ("Draw Mode")
      # "Multi-Band Mask Generation:\n\nCrafting the Multi-Band Mask for the left image.\nInverting the generated mask to obtain the corresponding mask for the right image."
      n75 = local read "ROI_X"() -> (w194:i32)
      n76 = local read "Wrapped Y"() -> (w202:i32)
      n77 = local read "X0"() -> (w198:dbl)
      n78 = Add(x=w198, y=0.0) -> (x+y=w199:dbl)
      n79 = Index Array(array=w197, index #1=7 ("index"), index #2=8 ("index")) -> (element #1=w203:T2, element #2=w215:T2)
      n80 = Build Array(0.0 ("element"), 0.0 ("element"), w198, w202) -> (w207:dbl[])
      n81 = call "IMAQ SetImageSize"("Y Resolution"=w202, "X Resolution"=w194, "Image"=w215) -> ("Image Out"=w214:T2)  [unwired: 2 in, 1 out]
      n82 = Build Array(w199, 0.0 ("element"), w194, w202) -> (w210:dbl[])
      n83 = call "IMAQ Draw"("Draw Mode"=w212, "Shape to draw"=w205, "Pixel Color"=sgl 1.0, "Coordinates"=w207, "Image Dst"=w214, "Image Src"=w214) -> ("Image Dst Out"=w211:T2)  [unwired: 4 in, 1 out]
      n84 = call "IMAQ Draw"("Draw Mode"=w212, "Shape to draw"=w205, "Pixel Color"=sgl 0.0, "Coordinates"=w210, "Image Dst"=w211, "Image Src"=w211) -> ("Image Dst Out"=w196:T2)  [unwired: 4 in, 1 out]
      n85 = call "IMAQ SetImageSize"("Y Resolution"=w202, "X Resolution"=w194, "Image"=w203) -> ("Image Out"=w204:T2)  [unwired: 2 in, 1 out]
      n86 = call "IMAQ Symmetry"("Type of Symmetry"=w201, "Image Dst"=w204, "Image Src"=w196) -> ("Image Dst Out"=w195:T2)  [unwired: 2 in, 1 out]
    }
    frame #8 {
      # "Establishing a designated space for memory storage (RGB)."
      n87 = for {
        N: 12 -> [_]
        tunnel: [w223] -> w219 mode=indexing
        i -> [w222]
        w224 = T11 4 items=["Grayscale (U8)", "Grayscale (I16)", "Grayscale (SGL)", "Complex (CSG)", "RGB (U32)", "HSL (U32)", "RGB (U64)", "Grayscale (U16)"] ("Image Type")
        n88 = Number To Decimal String(number=w222) -> (decimal integer string=w227:string)  [unwired: 1 out]
        n89 = Concatenate Strings("RGB" ("string"), w227) -> (w226:string)
        n90 = call "IMAQ Create"("Image Name"=w226, "Image Type"=w224) -> ("New Image"=w223:T2)  [unwired: 2 in, 2 out]
      }
    }
  }
  n91 = call <vilib>:"IMAQdx Open Camera.vi"("Session In"="Camera 2") -> ("error out"=w7:errorcluster, "Session Out"=w6:T3)  [unwired: 9 in]
  n92 = call <vilib>:"IMAQdx Open Camera.vi"("Session In"="Camera 1") -> ("error out"=w14:errorcluster, "Session Out"=w13:T3)  [unwired: 9 in]
  n93 = call <vilib>:"IMAQdx Configure Acquisition.vi"("error in"=w7, "Continuous?"=w2, "Session In"=w6) -> ("error out"=w10:errorcluster, "Session Out"=w11:T3)  [unwired: 7 in]
  n94 = call <vilib>:"IMAQdx Configure Acquisition.vi"("error in"=w14, "Continuous?"=w2, "Session In"=w13) -> ("error out"=w17:errorcluster, "Session Out"=w18:T3)  [unwired: 7 in]
  n95 = call <vilib>:"IMAQdx Enumerate Video Modes.vi"("error in"=w10, "Session In"=w11) -> ("error out"=w9:errorcluster, "Session Out"=w8:T3)  [unwired: 6 in, 2 out]
  n96 = call <vilib>:"IMAQdx Enumerate Video Modes.vi"("error in"=w17, "Session In"=w18) -> ("error out"=w16:errorcluster, "Session Out"=w15:T3)  [unwired: 6 in, 2 out]
  n97 = call <vilib>:"IMAQdx Start Acquisition.vi"("error in"=w9, "Session In"=w8) -> ("Session Out"=w3:T3)  [unwired: 8 in, 1 out]
  n98 = call <vilib>:"IMAQdx Start Acquisition.vi"("error in"=w16, "Session In"=w15) -> ("Session Out"=w4:T3)  [unwired: 8 in, 1 out]
  n99 = Build Array(w4, w3) -> (w1:T3[])
  n100 = while {
    tunnel: w21 -> [w243]
    tunnel: w29 -> [w242]
    tunnel: w28 -> [w241]
    tunnel: w30 -> [w240]
    tunnel: w26 -> [w239]
    tunnel: w27 -> [w238]
    tunnel: w25 -> [w237]
    tunnel: w24 -> [w236]
    tunnel: w23 -> [w235]
    tunnel: w22 -> [w234]
    tunnel: w20 -> [w233]
    tunnel: sgl[][] [[1.0, 2.0, 1.0], [2.0, 4.0, 2.0], [1.0, 2.0, 1.0]] ("Gaussian Kernel") -> [w232]
    tunnel: sgl[][] [[0.0, -1.0, 0.0], [-1.0, 4.0, -1.0], [0.0, -1.0, 0.0]] ("Laplace Kernel 2") -> [w231]
    tunnel: [w230] -> w34
    tunnel: [w229] -> w33
    tunnel: w1 -> [w228] mode=indexing
    stop <- "Stop" stop-if-true
    n101 = stacked-sequence {
      tunnel: w243 -> [_ _ _ _ _ _ _ _ _ _ _ _]
      tunnel: w242 -> [w248 _ w264 _ _ _ _ w357 w401 _ w792 _]
      tunnel: w241 -> [_ _ w263 _ _ _ _ _ _ _ _ _]
      tunnel: w240 -> [_ _ _ _ w298 _ _ w356 w402 _ _ _]
      tunnel: w239 -> [_ _ _ _ _ _ w342 _ _ _ _ _]
      tunnel: w238 -> [_ _ _ _ _ _ w341 _ _ _ _ _]
      tunnel: w237 -> [_ _ _ _ _ _ _ _ w394 _ _ _]
      tunnel: w236 -> [_ _ _ _ _ _ _ _ w393 _ _ _]
      tunnel: w235 -> [_ _ _ _ _ _ _ _ w400 _ _ _]
      tunnel: w234 -> [_ _ _ _ _ _ _ _ w399 _ _ _]
      tunnel: w233 -> [_ _ _ _ _ _ _ _ w398 _ _ _]
      tunnel: w232 -> [_ _ _ _ _ _ _ _ w397 _ _ _]
      tunnel: w231 -> [_ _ _ _ _ _ _ _ w396 _ _ _]
      tunnel: [_ _ _ _ _ _ _ _ _ _ w791 _] -> w230
      tunnel: [_ _ _ _ _ _ _ _ _ _ w790 _] -> w229
      tunnel: w228 -> [w246 _ _ _ _ _ _ _ _ _ _ _]
      frame #0 {
        # "Refining the Left and Right Image Acquisition Process:\n\nLoading the images.\nResizing the images to match the grid image size"
        n102 = Index Array(array=w248, index #1=0 ("index"), index #2=1 ("index")) -> (element #1=w252:T2, element #2=w251:T2)
        n103 = Build Array(w252, w251) -> (w247:T2[])
        n104 = for {
          tunnel: [w255] -> w245 mode=indexing
          tunnel: w247 -> [w259] mode=indexing
          tunnel: w246 -> [w257]
          tunnel: [w258] -> _ mode=indexing
          n105 = call <vilib>:"IMAQdx Calculate Frames per Second.vi"("Session In"=w257, "Buffer Number"=u32 0) -> ("Session Out"=w258:T3)  [unwired: 7 in, 6 out]
          n106 = call <vilib>:"IMAQdx Get Image2.vi"("Buffer Number Mode (Next)"=IMAQdx_Buffer_Number_Mode."Last New", "Image In"=w259, "Session In"=w257) -> ("Image Out"=w255:T2)  [unwired: 5 in, 3 out]
        }
        n107 = Index Array(array=w245) -> (element #1=→"Left Sample":T2, element #2=→"Right Sample":T2)  [unwired: 2 in]
      }
      frame #1 {
        # "Initiating time measurement for the system process."
        n108 = Get Date/Time In Seconds() -> (seconds since 1Jan1904=w262:timestamp)
        n109 = To Double Precision Float(number=w262) -> (double precision float=→"Start Time":dbl)
      }
      frame #2 {
        # "barrel Distortion Correction Process:\n\nTransferring calibration information on the captured images.\nRectifying lens distortion for both the left and right images"
        n110 = Index Array(array=w264, index #1=2 ("index"), index #2=3 ("index")) -> (element #1=w268:T2, element #2=w267:T2)
        n111 = Build Array(w268, w267) -> (w266:T2[])
        n112 = local read "Right Sample"() -> (w272:T2)
        n113 = local read "Left Sample"() -> (w273:T2)
        n114 = Build Array(w273, w272) -> (w271:T2[])
        n115 = for {
          tunnel: w271 -> [w276] mode=indexing
          tunnel: [w277] -> w265 mode=indexing
          tunnel: w266 -> [w275] mode=indexing
          tunnel: w263 -> [w274]
          n116 = call "IMAQ Set Calibration Info"("Image Dst"=w276, "Image Src"=w274) -> ("Calibrated Image"=w278:T2)  [unwired: 8 in, 1 out]
          n117 = call "IMAQ Correct Calibrated Image"("Image Dst"=w275, "Image Src"=w278) -> ("Corrected Image"=w277:T2)  [unwired: 8 in, 1 out]
        }
        "corrected" <- w265
      }
      frame #3 {
        # "Measuring the elapsed time for the barrel distortion correction process."
        n118 = local read "Start Time"() -> (w280:dbl)
        n119 = Get Date/Time In Seconds() -> (seconds since 1Jan1904=w282:timestamp)
        n120 = To Double Precision Float(number=w282) -> (double precision float=w281:dbl)
        "Correction End Time" <- w281
        n121 = Subtract(x=w281, y=w280) -> (x-y=→"Correction":dbl)
      }
      frame #4 {
        w291 = 0 items=["Polynomial"] ("Model")
        w288 = 0 items=["Polynomial", "Background Correction", "NiBlack"] ("Method")
        w299 = 5 ("Window Size")
        w320 = 5 items=["Red", "Green", "Blue", "Hue", "Saturation", "Luminance", "Value", "Intensity"] ("Color Plane")
        # "Flat Fielding Process:\n\nExtracting luminance planes for both images.\nMeasuring the SSIM factor.\nAveraging the luminance planes.\nEstimating the Master Flat Field plane.\nGenerating the flat-fielded planes.\nMeasuring the SSIM of the flat-fielded planes.\nReplacing the planes with the higher SSIM."
        n122 = Index Array(array=w298, index #1=9 ("index"), index #7=15 ("index")) -> (element #1=w318:T2, element #2=w317:T2, element #3=w315:T2, element #4=w309:T2, element #5=w308:T2, element #6=w305:T2, element #7=w304:T2)  [unwired: 5 in]
        n123 = local read "corrected"() -> (w293:T2[])
        n124 = Build Array(w318, w317) -> (w316:T2[])
        n125 = Build Array(w309, w308) -> (w307:T2[])
        n126 = Build Array(w305, w304) -> (w303:T2[])
        n127 = local read "corrected size"() -> (w283:cluster{"X Resolution":i32, "Y Resolution":i32})
        n128 = for {
          tunnel: w320 -> [w336]
          tunnel: w293 -> [w335] mode=indexing
          tunnel: w316 -> [w334] mode=indexing
          tunnel: [w333] -> w312 mode=indexing
          tunnel: [w333] -> w292 mode=indexing
          n129 = call "IMAQ ExtractSingleColorPlane"("Color Plane"=w336, "Image Dst"=w334, "Image Src"=w335) -> ("Image Dst Out"=w333:T2)  [unwired: 7 in, 1 out]
        }
        n130 = Bundle("Model"=w291, "corrected size"=w283, "Polynomial Degree"=1) -> (w284:T15)  [unwired: 1 in]
        n131 = Bundle("Estimate Background?"=TRUE, "Method"=w288, "Polynomial Degree"=1, "corrected size"=w283, "Niblack Deviation Factor (0.2)"=0.2) -> (w285:T16)  [unwired: 1 in]
        n132 = call "IMAQ Compute Average Image"("Image Dst"=w315, "Images"=w312) -> ("Image Dst Out"=w300:T2)  [unwired: 8 in, 1 out]
        n133 = Index Array(array=w292) -> (element #1=w314:T2, element #2=w313:T2)  [unwired: 2 in]
        n134 = for {
          tunnel: w292 -> [w330] mode=indexing
          tunnel: w300 -> [w332]
          tunnel: [w331] -> w296 mode=indexing
          tunnel: w307 -> [w328] mode=indexing
          tunnel: w303 -> [w327] mode=indexing
          tunnel: w284 -> [w326]
          tunnel: w285 -> [w325]
          n135 = call "IMAQ Estimate Flat Field Model"("Image Src"=w330, "Image Dst"=w328, "Mask Image"=w332, "Surface Fit Options"=w326, "Background Estimation Options"=w325) -> ("Flat Field Image Out"=w329:T2)  [unwired: 9 in, 1 out]
          n136 = call "IMAQ Flat Field Correction"("Image Src"=w330, "Image Dst"=w327, "Flat Field Image"=w329) -> ("Corrected Image"=w331:T2)  [unwired: 10 in, 2 out]
        }
        n137 = call-poly "IMAQ SSIM"("Window Size"=w299, "Reference Image"=w313, "Test Image"=w314) -> ("Mean SSIM"=w302:dbl)  [unwired: 4 in, 4 out]
        "SSIM Original" <- w302
        n138 = Index Array(array=w296) -> (element #1=w311:T2, element #2=w310:T2)  [unwired: 2 in]
        n139 = call-poly "IMAQ SSIM"("Window Size"=w299, "Reference Image"=w310, "Test Image"=w311) -> ("Mean SSIM"=w301:dbl)  [unwired: 4 in, 4 out]
        "SSIM Flat" <- w301
        n140 = Greater?(x=w302, y=w301) -> (0:w297:bool)
        "Original Luma?" <- w297
        n141 = Select(t=w292, s=w297, f=w296) -> (s? t:f=w295:T2[])
        n142 = for {
          tunnel: [w324] -> w294 mode=indexing
          tunnel: w293 -> [w323] mode=indexing
          tunnel: w295 -> [w322] mode=indexing
          w321 = u16 1 items=["RGB", "HSL", "HSV", "HSI"] ("Color Mode")
          n143 = call "IMAQ ReplaceColorPlane"("Image Src"=w323, "Color Mode"=w321, "Blue or Luma or Val or Inten Plane"=w322) -> ("Image Dst Out"=w324:T2)  [unwired: 11 in, 1 out]
        }
        "Adjusted" <- w294
      }
      frame #5 {
        # "Measuring the elapsed time for the Flat-Fielding process."
        n144 = local read "Correction End Time"() -> (w338:dbl)
        n145 = Get Date/Time In Seconds() -> (seconds since 1Jan1904=w340:timestamp)
        n146 = To Double Precision Float(number=w340) -> (double precision float=w339:dbl)
        "Flat Fielding End Time" <- w339
        n147 = Subtract(x=w339, y=w338) -> (x-y=→"Flat Fielding":dbl)
      }
      frame #6 {
        # "Image Wrapping:\n\nProjecting both the left and right images using the updated coordinates."
        n148 = Build Array(w341, w342) -> (w346:T2[])
        n149 = local read "Adjusted"() -> (w347:T2[])
        n150 = for {
          tunnel: w347 -> [w348] mode=indexing
          tunnel: w346 -> [w350] mode=indexing
          tunnel: [w349] -> w343 mode=indexing
          n151 = call "IMAQ Set Calibration Info"("Image Dst"=w348, "Image Src"=w350) -> ("Calibrated Image"=w351:T2)  [unwired: 8 in, 1 out]
          n152 = call "IMAQ Correct Calibrated Image"("Image Dst"=w348, "Image Src"=w351) -> ("Corrected Image"=w349:T2)  [unwired: 8 in, 1 out]
        }
        "Wrapped" <- w343
        n153 = Index Array(array=w343) -> (element #1=→"Left corrected, adjusted, and wrapped image":T2, element #2=→"Right corrected, adjusted, and wrapped image":T2)  [unwired: 2 in]
      }
      frame #7 {
        w387 = 0
        # "Region of Interest Extraction:\n\nIdentifying the ROIs in both left and right images.\nExtracting the RGB planes within the defined ROIs."
        n154 = Index Array(array=w357, index #1=4 ("index"), index #2=5 ("index")) -> (element #1=w378:T2, element #2=w377:T2)
        n155 = local read "Wrapped X"() -> (w352:i32)
        n156 = local read "ROI_X"() -> (w354:i32)
        n157 = Build Array(w378, w377) -> (w376:T2[])
        n158 = local read "Wrapped Y"() -> (w353:i32)
        n159 = Subtract(x=w352, y=w354) -> (x-y=w386:i32)
        n160 = Build Array(w387, w387, w354, w353) -> (w383:i32[])
        n161 = Build Array(w386, 0 ("element"), w352, w353) -> (w384:i32[])
        n162 = local read "Wrapped"() -> (w382:T2[])
        n163 = Build Array(w384, w383) -> (w381:i32[][])
        n164 = for {
          tunnel: w381 -> [w391] mode=indexing
          tunnel: [w388] -> _ mode=indexing
          tunnel: [w390] -> w360 mode=indexing
          tunnel: w376 -> [w389] mode=indexing
          tunnel: w382 -> [w388] mode=indexing
          n165 = call "IMAQ ColorImageToArray"("Optional Rectangle"=w391, "Image"=w388) -> ("Image Pixels (U32)"=w392:u32[][])  [unwired: 2 in, 2 out]
          n166 = call "IMAQ ArrayToColorImage"("Image Pixels (U32)"=w392, "Image"=w389) -> ("Image Out"=w390:T2)  [unwired: 3 in, 1 out]
        }
        n167 = Index Array(array=w360) -> (element #1=w362:T2, element #2=w361:T2)  [unwired: 2 in]
        "ROI_R" <- w361
        "ROI_L" <- w362
        n168 = Index Array(array=w356, index #1=16 ("index"), index #6=21 ("index")) -> (element #1=w374:T2, element #2=w373:T2, element #3=w372:T2, element #4=w371:T2, element #5=w370:T2, element #6=w369:T2)  [unwired: 4 in]
        n169 = call "IMAQ ExtractColorPlanes"("Blue or Luma or Val or Inten Plane"=w372, "Green or Sat Plane"=w373, "Red or Hue Plane"=w374, "Image Src"=w362) -> ("Blue or Luma or Val or Inten Plane out"=w366:T2, "Green or Sat Plane out"=w367:T2, "Red or Hue Plane out"=w368:T2)  [unwired: 4 in, 1 out]
        n170 = Build Array(w368, w367, w366) -> (→"RGB Left":T2[])
        n171 = call "IMAQ ExtractColorPlanes"("Blue or Luma or Val or Inten Plane"=w369, "Green or Sat Plane"=w370, "Red or Hue Plane"=w371, "Image Src"=w361) -> ("Blue or Luma or Val or Inten Plane out"=w363:T2, "Green or Sat Plane out"=w364:T2, "Red or Hue Plane out"=w365:T2)  [unwired: 4 in, 1 out]
        n172 = Build Array(w365, w364, w363) -> (→"RGB Right":T2[])
      }
      frame #8 {
        # "Blending the Regions Of Interest (ROIs) based on the chosen method."
        n173 = case shown="\"MBB\"" "Blending Method" {
          tunnel: w402 -> [w407 w472 w740]
          tunnel: w401 -> [w408 w471 w739]
          tunnel: w400 -> [w406 _ _]
          tunnel: w399 -> [w405 _ _]
          tunnel: w398 -> [_ w470 _]
          tunnel: w397 -> [_ w469 _]
          tunnel: w396 -> [_ w468 _]
          tunnel: [w404 w467 w738] -> w395
          tunnel: w394 -> [_ w466 _]
          tunnel: w393 -> [_ w465 _]
          frame "WA" {
            n174 = stacked-sequence {
              tunnel: w408 -> [w423]
              tunnel: w407 -> [w418]
              tunnel: w406 -> [w412]
              tunnel: w405 -> [w411]
              tunnel: [w419] -> w404
              frame #0 {
                # "Weighted Average Blending:\n\nComputing the weighted ROIs.\nCombining the weighted ROIs.\nAveraging the combined ROIs."
                n175 = call-poly <vilib>:"IMAQ ImageToEDVR.vi"("Image"=w411) -> ("EDVR 2D SGL"=w431:refnum<data-value>)  [unwired: 8 in, 2 out]
                n176 = Index Array(array=w418, index #1=22 ("index")) -> (element #1=w417:T2, element #2=w416:T2, element #3=w415:T2)  [unwired: 2 in]
                n177 = local read "RGB Right"() -> (w428:T2[])
                n178 = local read "RGB Left"() -> (w429:T2[])
                n179 = Build Array(w417, w416, w415) -> (w414:T2[])
                n180 = call-poly <vilib>:"IMAQ ImageToEDVR.vi"("Image"=w412) -> ("EDVR 2D SGL"=w430:refnum<data-value>)  [unwired: 8 in, 2 out]
                n181 = for {
                  tunnel: w428 -> [w440] mode=indexing
                  tunnel: w429 -> [w433] mode=indexing
                  tunnel: w430 -> [w438]
                  tunnel: w431 -> [w437]
                  tunnel: [w434] -> w427 mode=indexing
                  tunnel: w414 -> [w432] mode=indexing
                  n182 = call-poly <vilib>:"IMAQ ImageToEDVR.vi"("Image"=w440) -> ("EDVR 2D U8"=w441:refnum<data-value>)  [unwired: 8 in, 2 out]
                  n183 = call-poly <vilib>:"IMAQ ImageToEDVR.vi"("Image"=w433) -> ("EDVR 2D U8"=w439:refnum<data-value>)  [unwired: 8 in, 2 out]
                  n184 = in-place {
                    in-place-border: [w449] -> _
                    in-place-border: [w444] -> _
                    in-place-border: [w443] -> _
                    in-place-border: [w442] -> w435
                    n185 = in-place-dvr #1(w438) -> (w445:sgl[][])  [unwired: 1 out]
                    n186 = in-place-dvr #2(w437) -> (w446:sgl[][])  [unwired: 1 out]
                    n187 = in-place-dvr #3(w441) -> (w447:u8[][])  [unwired: 1 out]
                    n188 = in-place-dvr #4(w439) -> (w448:u8[][])  [unwired: 1 out]
                    n189 = for {
                      tunnel: w447 -> [w457] mode=indexing
                      workers-P: _ -> [_]
                      tunnel: [w456] -> w449 mode=indexing
                      tunnel: w448 -> [w455] mode=indexing
                      tunnel: w446 -> [w454] mode=indexing
                      tunnel: w445 -> [w453] mode=indexing
                      tunnel: [w452] -> w444 mode=indexing
                      tunnel: [w451] -> w443 mode=indexing
                      tunnel: [w450] -> w442 mode=indexing
                      n190 = for {
                        tunnel: w457 -> [w464] mode=indexing
                        tunnel: [w460] -> w456 mode=indexing
                        tunnel: w455 -> [w458] mode=indexing
                        tunnel: w453 -> [w459] mode=indexing
                        tunnel: w454 -> [w463] mode=indexing
                        tunnel: [w462] -> w452 mode=indexing
                        tunnel: [w461] -> w450 mode=indexing
                        tunnel: [w460] -> w451 mode=indexing
                        n191 = Multiply(x=w458, y=w459) -> (x*y=w462:sgl)
                        n192 = Multiply(x=w464, y=w463) -> (x*y=w460:sgl)
                        n193 = Add(x=w460, y=w462) -> (x+y=w461:sgl)
                      }
                    }
                    n194 = in-place-dvr #1(w445) -> ()  [unwired: 2 out]
                    n195 = in-place-dvr #2(w446) -> ()  [unwired: 2 out]
                    n196 = in-place-dvr #3(w447) -> ()  [unwired: 2 out]
                    n197 = in-place-dvr #4(w448) -> ()  [unwired: 2 out]
                  }
                  n198 = To Unsigned Byte Integer(number=w435) -> (unsigned 8bit integer=w436:u8[][])
                  n199 = call "IMAQ ArrayToImage"("Image Pixels (U8)"=w436, "Image"=w432) -> ("Image Out"=w434:T2)  [unwired: 8 in, 1 out]
                }
                n200 = local read "Wrapped Y"() -> (w410:i32)
                n201 = Index Array(array=w423, index=6) -> (element=w421:T2)
                n202 = local read "ROI_X"() -> (w409:i32)
                n203 = call "IMAQ SetImageSize"("Y Resolution"=w410, "X Resolution"=w409, "Image"=w421) -> ("Image Out"=w420:T2)  [unwired: 2 in, 1 out]
                n204 = Index Array(array=w427) -> (element #1=w426:T2, element #2=w425:T2, element #3=w424:T2)  [unwired: 3 in]
                n205 = call "IMAQ ReplaceColorPlane"("Image Src"=w420, "Red or Hue Plane"=w426, "Green or Sat Plane"=w425, "Blue or Luma or Val or Inten Plane"=w424) -> ("Image Dst Out"=w419:T2)  [unwired: 10 in, 1 out]
              }
            }
          }
          frame "MBB" {
            n206 = stacked-sequence {
              tunnel: w472 -> [w476 w502 w552 _ w664 w705]
              tunnel: w471 -> [_ _ _ w614 w665 w703]
              tunnel: w470 -> [_ w501 w554 _ _ w704]
              tunnel: w469 -> [_ w500 _ _ _ _]
              tunnel: w468 -> [_ _ w553 _ _ _]
              tunnel: [_ _ _ _ _ w702] -> w467
              tunnel: w466 -> [w474 _ _ _ _ _]
              tunnel: w465 -> [w475 _ _ _ _ _]
              frame #0 {
                # "Multi-Band Blending:\n\nMasking the ROIs.\nGenerating the Gaussian Pyramid of the masked ROIs.\nGenerating the Laplacian Pyramid of the ROIs.\nBlending the Pyramids starting from the lowest resolution."
                n207 = Index Array(array=w476, index #1=25 ("index"), index #6=30 ("index")) -> (element #1=w487:T2, element #2=w486:T2, element #3=w485:T2, element #4=w483:T2, element #5=w482:T2, element #6=w481:T2)  [unwired: 4 in]
                n208 = local read "RGB Right"() -> (w477:T2[])
                n209 = local read "RGB Left"() -> (w478:T2[])
                n210 = Build Array(w487, w486, w485) -> (w484:T2[])
                n211 = Build Array(w483, w482, w481) -> (w480:T2[])
                n212 = for {
                  tunnel: w478 -> [w497] mode=indexing
                  tunnel: w477 -> [w496] mode=indexing
                  tunnel: [w495] -> w489 mode=indexing
                  tunnel: [w494] -> w488 mode=indexing
                  tunnel: w484 -> [w493] mode=indexing
                  tunnel: w480 -> [w492] mode=indexing
                  tunnel: w475 -> [w491]
                  tunnel: w474 -> [w490]
                  n213 = call "IMAQ Multiply"("Image Src A"=w496, "Image Dst"=w492, "Image Src B"=w490) -> ("Image Dst Out"=w495:T2)  [unwired: 4 in, 1 out]
                  n214 = call "IMAQ Multiply"("Image Src A"=w497, "Image Dst"=w493, "Image Src B"=w491) -> ("Image Dst Out"=w494:T2)  [unwired: 4 in, 1 out]
                }
                "Masked RGB Right MBB" <- w489
                "Masked RGB Left MBB" <- w488
              }
              frame #1 {
                w513 = 6 ("length")
                w520 = 31 ("index")
                n215 = Array Subset(array=w502, index=w520, length=w513) -> (w524:T2[])
                n216 = Add(x=w520, y=w513) -> (x+y=w519:i32)
                n217 = Array Subset(array=w502, index=w519, length=w513) -> (w523:T2[])
                n218 = Add(x=w519, y=w513) -> (x+y=w518:i32)
                n219 = Array Subset(array=w502, index=w518, length=w513) -> (w522:T2[])
                n220 = Add(x=w518, y=w513) -> (x+y=w517:i32)
                n221 = Array Subset(array=w502, index=w517, length=w513) -> (w521:T2[])
                n222 = Add(x=w517, y=w513) -> (x+y=w516:i32)
                n223 = Array Subset(array=w502, index=w516, length=w513) -> (w511:T2[])
                n224 = Add(x=w516, y=w513) -> (x+y=w515:i32)
                n225 = Array Subset(array=w502, index=w515, length=w513) -> (w510:T2[])
                n226 = Add(x=w515, y=w513) -> (x+y=w514:i32)
                n227 = local read "Wrapped X"() -> (w498:i32)
                n228 = local read "Wrapped Y"() -> (w499:i32)
                n229 = Add(x=w514, y=w513) -> (x+y=w512:i32)
                n230 = Array Subset(array=w502, index=w514, length=w513) -> (w509:T2[])
                n231 = local read "Masked RGB Right MBB"() -> (w505:T2[])
                n232 = local read "Masked RGB Left MBB"() -> (w506:T2[])
                n233 = local read "Y0"() -> (w529:dbl)
                n234 = local read "Y1"() -> (w528:dbl)
                n235 = local read "Y2"() -> (w527:dbl)
                n236 = local read "X0"() -> (w532:dbl)
                n237 = local read "X1"() -> (w531:dbl)
                n238 = local read "X2"() -> (w530:dbl)
                n239 = Array Subset(array=w502, index=w512, length=w513) -> (w508:T2[])
                n240 = Build Array(w499, w529, w528, w527) -> (w525:dbl[])
                n241 = Build Array(w498, w532, w531, w530) -> (w526:dbl[])
                n242 = Build Array(w524, w523, w522, w521, w511, w510, w509, w508) -> (w507:T2[][])
                n243 = Insert Into Array(array=w506, new element=w505) -> (w504:T2[])  [unwired: 1 in]
                n244 = for {
                  tunnel: w526 -> [w540] mode=indexing
                  tunnel: w525 -> [w539] mode=indexing
                  tunnel: [w538] -> w503 mode=indexing
                  tunnel: w500 -> [w537]
                  tunnel: w507 -> [w535] mode=indexing
                  tunnel: w501 -> [w533]
                  tunnel: w504 -> [w534]
                  n245 = for {
                    N: 6 -> [_]
                    tunnel: w534 -> [w548] mode=indexing
                    tunnel: w540 -> [w547]
                    tunnel: w539 -> [w546]
                    tunnel: [w545] -> w538 mode=indexing
                    tunnel: w537 -> [w544]
                    tunnel: w535 -> [w543] mode=indexing
                    tunnel: w533 -> [w541]
                    n246 = call "IMAQ Convolute"("Kernel"=w544, "Image Src"=w548) -> ("error out"=w549:errorcluster, "Image Dst Out"=w542:T2)  [unwired: 8 in]
                    n247 = call "IMAQ Resample"("X Resolution"=w547, "Y Resolution"=w546, "error in (no error)"=w549, "Interpolation Type"=w541, "Image Dst"=w543, "Image Src"=w542) -> ("Image Dst Out"=w545:T2)  [unwired: 4 in, 1 out]
                  }
                }
                "GP" <- w503
              }
              frame #2 {
                w571 = 6 ("length")
                w578 = 55 ("index")
                n248 = Array Subset(array=w552, index=w578, length=w571) -> (w582:T2[])
                n249 = Add(x=w578, y=w571) -> (x+y=w577:i32)
                n250 = Array Subset(array=w552, index=w577, length=w571) -> (w581:T2[])
                n251 = Add(x=w577, y=w571) -> (x+y=w576:i32)
                n252 = Array Subset(array=w552, index=w576, length=w571) -> (w580:T2[])
                n253 = Add(x=w576, y=w571) -> (x+y=w575:i32)
                n254 = Array Subset(array=w552, index=w575, length=w571) -> (w579:T2[])
                n255 = Add(x=w575, y=w571) -> (x+y=w574:i32)
                n256 = Array Subset(array=w552, index=w574, length=w571) -> (w569:T2[])
                n257 = Add(x=w574, y=w571) -> (x+y=w573:i32)
                n258 = local read "Wrapped Y"() -> (w550:i32)
                n259 = local read "ROI_X"() -> (w551:i32)
                n260 = Array Subset(array=w552, index=w573, length=w571) -> (w568:T2[])
                n261 = Add(x=w573, y=w571) -> (x+y=w572:i32)
                n262 = local read "X0"() -> (w586:dbl)
                n263 = local read "X1"() -> (w585:dbl)
                n264 = local read "Y0"() -> (w584:dbl)
                n265 = local read "Y1"() -> (w583:dbl)
                n266 = Add(x=w572, y=w571) -> (x+y=w570:i32)
                n267 = Array Subset(array=w552, index=w572, length=w571) -> (w567:T2[])
                n268 = Build Array(w550, w584, w583) -> (w561:dbl[])
                n269 = Build Array(w551, w586, w585) -> (w563:dbl[])
                n270 = local read "GP"() -> (w559:T2[][])
                n271 = Array Subset(array=w552, index=w570, length=w571) -> (w566:T2[])
                n272 = Reshape Array(w559, 24 ("dimension size")) -> (w558:T2[])
                n273 = Build Array(w582, w581, w580, w579, w569, w568, w567, w566) -> (w565:T2[][])
                n274 = Reverse 1D Array(array=w563) -> (reversed array=w562:dbl[])
                n275 = Reverse 1D Array(array=w561) -> (reversed array=w560:dbl[])
                n276 = Reverse 1D Array(array=w558) -> (reversed array=w557:T2[])
                n277 = for {
                  tunnel: w562 -> [w595] mode=indexing
                  tunnel: w560 -> [w594] mode=indexing
                  tunnel: [w593] -> w564 mode=indexing
                  tunnel: w553 -> [w592]
                  tunnel: w565 -> [w590] mode=indexing
                  tunnel: w554 -> [w589]
                  tunnel: w557 -> [w588]
                  tunnel: sgl 15.0 ("Divider (kernel sum)") -> [w587]
                  n278 = for {
                    N: 6 -> [_]
                    tunnel: w588 -> [w600] mode=indexing
                    tunnel: w595 -> [w604]
                    tunnel: w594 -> [w603]
                    tunnel: [w598] -> w593 mode=indexing
                    tunnel: w592 -> [w597]
                    tunnel: w590 -> [w602] mode=indexing
                    tunnel: w589 -> [w601]
                    tunnel: w587 -> [w596]
                    n279 = call "IMAQ Resample"("X Resolution"=w604, "Y Resolution"=w603, "Interpolation Type"=w601, "Image Dst"=w602, "Image Src"=w600) -> ("Image Dst Out"=w599:T2)  [unwired: 5 in, 1 out]
                    n280 = call "IMAQ Convolute"("Kernel"=w597, "Divider (kernel sum)"=w596, "Image Src"=w599) -> ("Image Dst Out"=w598:T2)  [unwired: 7 in, 1 out]
                  }
                }
                "LP" <- w564
              }
              frame #3 {
                n281 = local read "GP"() -> (w630:T2[][])
                n282 = local read "LP"() -> (w644:T2[][])
                n283 = Array Subset(array=w644, index (row)=0 ("index"), length (row)=3 ("length"), index (col)=0 ("index"), length (col)=3 ("length")) -> (w636:T2[][])
                n284 = Array Subset(array=w644, index (row)=0 ("index"), length (row)=3 ("length"), index (col)=3 ("index"), length (col)=3 ("length")) -> (w635:T2[][])
                n285 = Array Subset(array=w630, index (row)=0 ("index"), length (row)=3 ("length"), index (col)=0 ("index"), length (col)=3 ("length")) -> (w625:T2[][])
                n286 = Array Subset(array=w630, index (row)=0 ("index"), length (row)=3 ("length"), index (col)=3 ("index"), length (col)=3 ("length")) -> (w624:T2[][])
                n287 = for {
                  tunnel: w636 -> [w657] mode=indexing
                  tunnel: w635 -> [w656] mode=indexing
                  tunnel: [w652] -> w620 mode=indexing
                  tunnel: w625 -> [w655] mode=indexing
                  tunnel: w624 -> [w654] mode=indexing
                  tunnel: [w653] -> w613 mode=indexing
                  n288 = for {
                    tunnel: w657 -> [w663] mode=indexing
                    tunnel: w656 -> [w662] mode=indexing
                    tunnel: [w661] -> w653 mode=indexing
                    tunnel: w655 -> [w660] mode=indexing
                    tunnel: w654 -> [w659] mode=indexing
                    tunnel: [w658] -> w652 mode=indexing
                    n289 = call "IMAQ Add"("Image Src A"=w663, "Image Src B"=w662) -> ("Image Dst Out"=w661:T2)  [unwired: 5 in, 1 out]
                    n290 = call "IMAQ Add"("Image Src A"=w660, "Image Src B"=w659) -> ("Image Dst Out"=w658:T2)  [unwired: 5 in, 1 out]
                  }
                }
                "Combined Laplace" <- w613
                n291 = Array Subset(array=w613, index (row)=0 ("index"), length (row)=3 ("length")) -> (w619:T2[][])  [unwired: 2 in]
                n292 = Array Subset(array=w620, index (row)=2 ("index")) -> (w618:T2[][])  [unwired: 3 in]
                n293 = for {
                  tunnel: w619 -> [w648] mode=indexing
                  tunnel: w618 -> [w647] mode=indexing
                  tunnel: [w646] -> w616 mode=indexing
                  n294 = for {
                    tunnel: w648 -> [w651] mode=indexing
                    tunnel: w647 -> [w650] mode=indexing
                    tunnel: [w649] -> w646 mode=indexing
                    n295 = call "IMAQ Add"("Image Src A"=w651, "Image Src B"=w650) -> ("Image Dst Out"=w649:T2)  [unwired: 5 in, 1 out]
                  }
                }
                n296 = Index Array(array=w614, index=7) -> (element=w612:T2)
                n297 = local read "X1"() -> (w606:dbl)
                n298 = local read "Y1"() -> (w605:dbl)
                n299 = Reshape Array(w616, 3 ("dimension size")) -> (w607:T2[])
                n300 = call "IMAQ SetImageSize"("Y Resolution"=w605, "X Resolution"=w606, "Image"=w612) -> ("Image Out"=w611:T2)  [unwired: 2 in, 1 out]
                n301 = Index Array(array=w607) -> (element #1=w610:T2, element #2=w609:T2, element #3=w608:T2)  [unwired: 3 in]
                n302 = call "IMAQ ReplaceColorPlane"("Image Src"=w611, "Red or Hue Plane"=w610, "Green or Sat Plane"=w609, "Blue or Luma or Val or Inten Plane"=w608) -> ()  [unwired: 10 in, 2 out]
              }
              frame #4 {
                w684 = u16 0 items=["RGB", "HSL", "HSV", "HSI"] ("Color Mode")
                n303 = Index Array(array=w664, index #1=80 ("index")) -> (element #1=w687:T2, element #2=w686:T2, element #3=w685:T2)  [unwired: 2 in]
                n304 = Index Array(array=w665, index=7) -> (element=w666:T2)
                n305 = local read "Combined Laplace"() -> (w683:T2[][])
                n306 = call "IMAQ ExtractColorPlanes"("Blue or Luma or Val or Inten Plane"=w685, "Color Mode"=w684, "Green or Sat Plane"=w686, "Red or Hue Plane"=w687, "Image Src"=w666) -> ("Blue or Luma or Val or Inten Plane out"=w690:T2, "Green or Sat Plane out"=w691:T2, "Red or Hue Plane out"=w692:T2)  [unwired: 3 in, 1 out]
                n307 = local read "Correction Interpolation"() -> (w668:u32)
                n308 = Array Subset(array=w683, index (row)=1 ("index"), length (row)=1 ("length")) -> (w680:T2[][])  [unwired: 2 in]
                n309 = Build Array(w692, w691, w690) -> (w689:T2[])
                n310 = local read "X0"() -> (w675:dbl)
                n311 = local read "Y0"() -> (w674:dbl)
                n312 = Index Array(array=w665, index=8) -> (element=w676:T2)
                n313 = Reshape Array(w680, 3 ("dimension size")) -> (w678:T2[])
                n314 = for {
                  tunnel: w689 -> [w697] mode=indexing
                  tunnel: w675 -> [w699]
                  tunnel: w674 -> [w698]
                  tunnel: [w694] -> w672 mode=indexing
                  tunnel: w678 -> [w695] mode=indexing
                  tunnel: w668 -> [w693]
                  n315 = call "IMAQ Resample"("X Resolution"=w699, "Y Resolution"=w698, "Interpolation Type"=w693, "Image Src"=w697) -> ("Image Dst Out"=w696:T2)  [unwired: 6 in, 1 out]
                  n316 = call "IMAQ Add"("Image Src A"=w696, "Image Src B"=w695) -> ("Image Dst Out"=w694:T2)  [unwired: 5 in, 1 out]
                }
                n317 = call "IMAQ SetImageSize"("Y Resolution"=w674, "X Resolution"=w675, "Image"=w676) -> ("Image Out"=w673:T2)  [unwired: 2 in, 1 out]
                n318 = Index Array(array=w672) -> (element #1=w669:T2, element #2=w670:T2, element #3=w671:T2)  [unwired: 3 in]
                n319 = call "IMAQ ReplaceColorPlane"("Image Src"=w673, "Red or Hue Plane"=w669, "Green or Sat Plane"=w670, "Blue or Luma or Val or Inten Plane"=w671) -> ()  [unwired: 10 in, 2 out]
              }
              frame #5 {
                w721 = u16 0 items=["RGB", "HSL", "HSV", "HSI"] ("Color Mode")
                n320 = Index Array(array=w705, index #1=83 ("index")) -> (element #1=w724:T2, element #2=w723:T2, element #3=w722:T2)  [unwired: 2 in]
                n321 = Index Array(array=w703, index=8) -> (element=w706:T2)
                n322 = local read "Combined Laplace"() -> (w720:T2[][])
                n323 = call "IMAQ ExtractColorPlanes"("Blue or Luma or Val or Inten Plane"=w722, "Color Mode"=w721, "Green or Sat Plane"=w723, "Red or Hue Plane"=w724, "Image Src"=w706) -> ("Blue or Luma or Val or Inten Plane out"=w727:T2, "Green or Sat Plane out"=w728:T2, "Red or Hue Plane out"=w729:T2)  [unwired: 3 in, 1 out]
                n324 = Array Subset(array=w720, index (row)=2 ("index"), length (row)=1 ("length")) -> (w717:T2[][])  [unwired: 2 in]
                n325 = local read "Wrapped Y"() -> (w700:i32)
                n326 = local read "ROI_X"() -> (w701:i32)
                n327 = Build Array(w729, w728, w727) -> (w726:T2[])
                n328 = Index Array(array=w703, index=9) -> (element=w713:T2)
                n329 = Reshape Array(w717, 3 ("dimension size")) -> (w715:T2[])
                n330 = for {
                  tunnel: w726 -> [w735] mode=indexing
                  tunnel: w701 -> [w736]
                  tunnel: w700 -> [w730]
                  tunnel: [w734] -> w708 mode=indexing
                  tunnel: w715 -> [w732] mode=indexing
                  tunnel: w704 -> [w731]
                  tunnel: w701 -> [_]
                  n331 = call "IMAQ Resample"("X Resolution"=w736, "Y Resolution"=w730, "Interpolation Type"=w731, "Image Src"=w735) -> ("Image Dst Out"=w733:T2)  [unwired: 6 in, 1 out]
                  n332 = call "IMAQ Add"("Image Src A"=w733, "Image Dst"=w732, "Image Src B"=w732) -> ("Image Dst Out"=w734:T2)  [unwired: 4 in, 1 out]
                }
                n333 = call "IMAQ SetImageSize"("Y Resolution"=w700, "X Resolution"=w701, "Image"=w713) -> ("Image Out"=w712:T2)  [unwired: 2 in, 1 out]
                n334 = Index Array(array=w708) -> (element #1=w709:T2, element #2=w710:T2, element #3=w711:T2)  [unwired: 3 in]
                n335 = call "IMAQ ReplaceColorPlane"("Image Src"=w712, "Red or Hue Plane"=w709, "Green or Sat Plane"=w710, "Blue or Luma or Val or Inten Plane"=w711) -> ("Image Dst Out"=w702:T2)  [unwired: 10 in, 1 out]
              }
            }
          }
          frame "WE" {
            w743 = u16 0 items=["RGB", "HSL", "HSV", "HSI"] ("Color Mode")
            # "Wavelet Extraction Blending:\n\nApplying the Haar filter on the ROIs.\nExtracting the low frequencies.\nCombining and scaling the low frequencies of the ROIs."
            n336 = Index Array(array=w740, index #1=86 ("index")) -> (element #1=w753:T2, element #2=w752:T2, element #3=w751:T2)  [unwired: 2 in]
            n337 = local read "Original Luma?"() -> (w754:bool)
            n338 = Build Array(w753, w752, w751) -> (w758:T2[])
            n339 = case shown="True" w754 {
              tunnel: [w760 w764] -> w755
              frame False {
                n340 = local read "SSIM Flat"() -> (w763:dbl)
                n341 = Multiply(x=w763, y=10.0) -> (x*y=w761:dbl)
                n342 = Round Toward +Infinity(x=w761) -> (ceil(x): smallest int >= x=w760:dbl)
              }
              frame True {
                n343 = local read "SSIM Original"() -> (w767:dbl)
                n344 = Multiply(x=w767, y=10.0) -> (x*y=w765:dbl)
                n345 = Round Toward +Infinity(x=w765) -> (ceil(x): smallest int >= x=w764:dbl)
              }
            }
            n346 = local read "RGB Right"() -> (w757:T2[])
            n347 = local read "RGB Left"() -> (w756:T2[])
            n348 = for {
              tunnel: w758 -> [w780] mode=indexing
              tunnel: [w768] -> w746
              tunnel: w755 -> [w774]
              tunnel: w756 -> [w777] mode=indexing
              tunnel: w757 -> [w776] mode=indexing
              tunnel: [w768] -> w759 mode=indexing
              n349 = call "IMAQ Extract Wavelet Bands"("Image"=w777) -> ("LL"=w779:sgl[][], "HH"=w773:sgl[][])  [unwired: 6 in, 7 out]
              n350 = call "IMAQ Extract Wavelet Bands"("Image"=w776) -> ("LL"=w778:sgl[][], "HH"=w772:sgl[][])  [unwired: 6 in, 7 out]
              n351 = Add(x=w779, y=w778) -> (x+y=w771:sgl[][])
              n352 = Add(x=w773, y=w772) -> (x+y=w770:sgl[][])
              n353 = Add(x=w771, y=w770) -> (x+y=w769:sgl[][])
              n354 = Divide(x=w769, y=w774) -> (x/y=w775:dbl[][])
              n355 = call "IMAQ ArrayToImage"("Image Pixels (U8)"=w775, "Image"=w780) -> ("Image Out"=w768:T2)  [unwired: 8 in, 1 out]
            }
            n356 = Index Array(array=w739, index=10) -> (element=w737:T2)
            n357 = call "IMAQ GetImageInfo"("Image"=w746) -> ("Y Resolution"=w744:i32, "X Resolution"=w745:i32)  [unwired: 3 in, 6 out]
            n358 = call "IMAQ SetImageSize"("Y Resolution"=w744, "X Resolution"=w745, "Image"=w737) -> ("Image Out"=w750:T2)  [unwired: 2 in, 1 out]
            n359 = Index Array(array=w759) -> (element #1=w749:T2, element #2=w748:T2, element #3=w747:T2)  [unwired: 3 in]
            n360 = call "IMAQ ReplaceColorPlane"("Image Src"=w750, "Color Mode"=w743, "Red or Hue Plane"=w749, "Green or Sat Plane"=w748, "Blue or Luma or Val or Inten Plane"=w747) -> ("Image Dst Out"=w738:T2)  [unwired: 9 in, 1 out]
          }
        }
        "Blended ROI" <- w395
      }
      frame #9 {
        # "Measuring the elapsed time for the blending process."
        n361 = local read "Flat Fielding End Time"() -> (w782:dbl)
        n362 = Get Date/Time In Seconds() -> (seconds since 1Jan1904=w784:timestamp)
        n363 = To Double Precision Float(number=w784) -> (double precision float=w783:dbl)
        "Blending End Time" <- w783
        n364 = Subtract(x=w783, y=w782) -> (x-y=→"ROI Blending":dbl)
      }
      frame #10 {
        w795 = 0 ("element")
        # "Panorama Generation:\n\nCreating the panorama destination.\nSetting the size based on the entire images' sizes.\nPositioning the left and right images.\nPositioning the blended ROI.\nProjecting the images onto the panorama destination."
        n365 = local read "Blended ROI"() -> (w789:T2)
        n366 = local read "Wrapped X"() -> (w786:i32)
        n367 = local read "Wrapping Factor"() -> (w800:i32)
        n368 = local read "ROI_X"() -> (w788:i32)
        n369 = Multiply(x=w786, y=2) -> (x*y=w810:i32)
        n370 = local read "Left corrected, adjusted, and wrapped image"() -> (w806:T2)
        n371 = Index Array(array=w792, index=11) -> (element=w811:T2)
        n372 = local read "Wrapped Y"() -> (w787:i32)
        n373 = Subtract(x=w786, y=w788) -> (x-y=w804:i32)
        n374 = Subtract(x=w810, y=w788) -> (x-y=w798:i32)
        n375 = Less Or Equal?(x=w800, y=7) -> (x <= y?=w801:bool)
        n376 = local read "Right corrected, adjusted, and wrapped image"() -> (w805:T2)
        n377 = case shown="False" w801 {
          tunnel: w798 -> [w815 w828]
          tunnel: w800 -> [w814 w826]
          tunnel: [w813 w827] -> w785
          tunnel: w787 -> [w812 w824]
          frame True {
            n378 = Subtract(x=7, y=w814) -> (x-y=w820:i32)
            n379 = Multiply(x=w820, y=7) -> (x*y=w821:i32)
            n380 = Add(x=20 ("y"), y=w821) -> (x+y=w822:i32)
            n381 = Subtract(x=w812, y=w822) -> (x-y=w823:i32)
            n382 = Build Array(0.0 ("element"), w822, w815, w823) -> (w813:dbl[])
          }
          frame False {
            n383 = Subtract(x=w826, y=8) -> (x-y=w832:i32)
            n384 = Multiply(x=w832, y=5) -> (x*y=w833:i32)
            n385 = Subtract(x=32 ("y"), y=w833) -> (x-y=w834:i32)
            n386 = Subtract(x=w824, y=w834) -> (x-y=w835:i32)
            n387 = Build Array(0.0 ("element"), w834, w828, w835) -> (w827:dbl[])
          }
        }
        n388 = call "IMAQ SetImageSize"("Y Resolution"=w787, "X Resolution"=w798, "Image"=w811) -> ("Image Out"=w809:T2)  [unwired: 2 in, 1 out]
        n389 = Build Array(0.0 ("element"), w795) -> (w802:dbl[])
        n390 = call "IMAQ ImageToImage 2"("Offset Left/Top"=w802, "Image Src (Small)"=w806, "Image Src (Large)"=w809) -> ("Image Dst Out"=w808:T2)  [unwired: 7 in, 1 out]
        n391 = Build Array(w804, w795) -> (w803:i32[])
        n392 = call "IMAQ ImageToImage 2"("Offset Left/Top"=w803, "Image Src (Small)"=w805, "Image Src (Large)"=w808) -> ("Image Dst Out"=w807:T2)  [unwired: 7 in, 1 out]
        n393 = call "IMAQ ImageToImage 2"("Offset Left/Top"=w803, "Image Src (Small)"=w789, "Image Src (Large)"=w807) -> ("Image Dst Out"=w799:T2)  [unwired: 7 in, 1 out]
        n394 = call "IMAQ Extract 2"("Optional Rectangle"=w785, "Image Src"=w799) -> ("error out"=w790:errorcluster, "Image Dst Out"=w791:T2)  [unwired: 8 in]
        "Panorama Image" <- w791
      }
      frame #11 {
        # "Calculating the Frames Per Second (FPS) for the processed output."
        n395 = local read "Start Time"() -> (w839:dbl)
        n396 = Get Date/Time In Seconds() -> (seconds since 1Jan1904=w841:timestamp)
        n397 = To Double Precision Float(number=w841) -> (double precision float=w840:dbl)
        n398 = Subtract(x=w840, y=w839) -> (x-y=w837:dbl)
        n399 = Divide(x=1.0, y=w837) -> (x/y=→"Processed FPS":dbl)
      }
    }
  }
  n400 = call "IMAQ Dispose"("Image"=w34, "error in (no error)"=w33) -> ("error out"=→"error out":errorcluster)  [unwired: 4 in]
